vi "_API_BINANCE_GET_USDT_FUTURES_AccountInformation.vi"(0 "BinanceAPI in":refnum<class "BinanceAPI_.lvclass">, 11 "error in (no error)":errorcluster) -> (4 "BinanceAPI out":refnum<class "BinanceAPI_.lvclass">, 6 "data":T1, 14 "Data":string, 15 "error out":errorcluster)   [LabVIEW 2022 SP3, in "BinanceAPI_.lvclass"]
uses:
  BinanceAPI_.lvclass
  BinanceAPI_.lvclass/BinanceAPI_.ctl
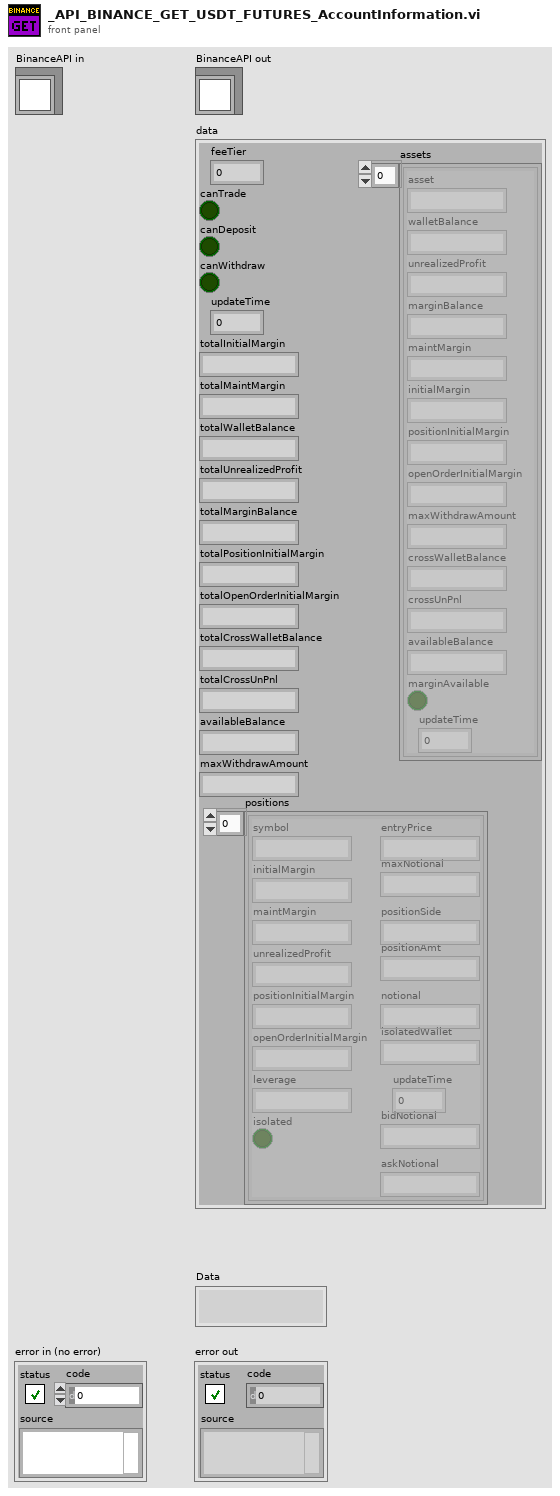
[diagram p1: front panel]
types:
  T1 = cluster{"feeTier":dbl, "canTrade":bool, "canDeposit":bool, "canWithdraw":bool, "updateTime":dbl, "totalInitialMargin":string, "totalMaintMargin":string, "totalWalletBalance":string, "totalUnrealizedProfit":string, "totalMarginBalance":string, "totalPositionInitialMargin":string, "totalOpenOrderInitialMargin":string, "totalCrossWalletBalance":string, "totalCrossUnPnl":string, "availableBalance":string, "maxWithdrawAmount":string, "assets":cluster{"asset":string, "walletBalance":string, "unrealizedProfit":string, "marginBalance":string, "maintMargin":string, "initialMargin":string, "positionInitialMargin":string, "openOrderInitialMargin":string, "maxWithdrawAmount":string, "crossWalletBalance":string, "crossUnPnl":string, "availableBalance":string, "marginAvailable":bool, "updateTime":dbl}[], "positions":cluster{"symbol":string, "initialMargin":string, "maintMargin":string, "unrealizedProfit":string, "positionInitialMargin":string, "openOrderInitialMargin":string, "leverage":string, "isolated":bool, "entryPrice":string, "maxNotional":string, "positionSide":string, "positionAmt":string, "notional":string, "isolatedWallet":string, "updateTime":dbl, "bidNotional":string, "askNotional":string}[]}
  T2 = enum16{"SPOT", "USDT_FUTURES", "COIN_FUTURES", "VANILLA"}
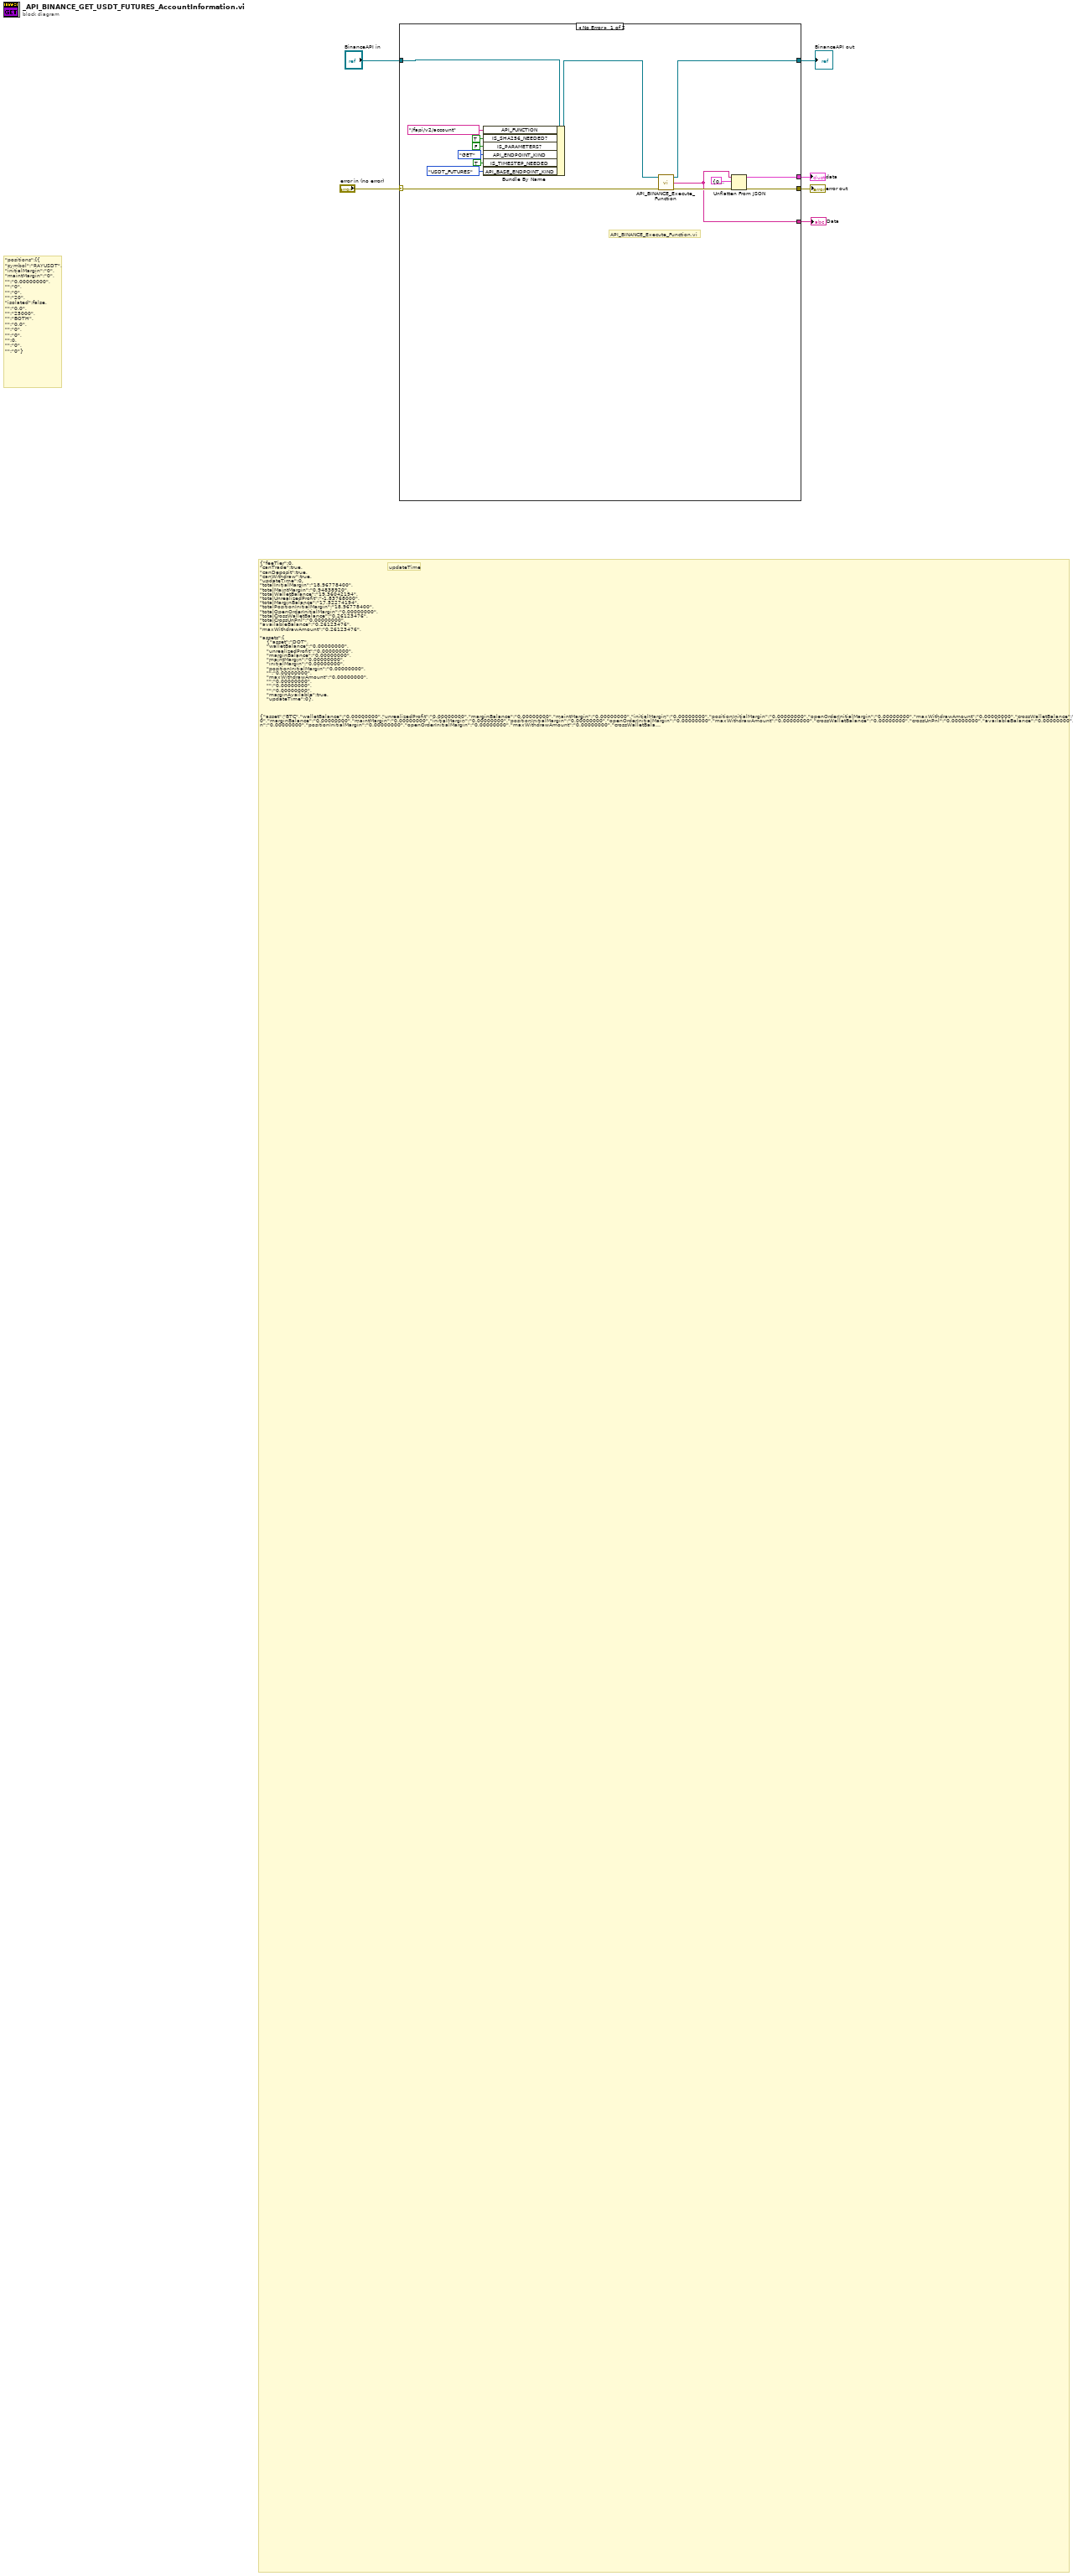
[diagram p0: block diagram]
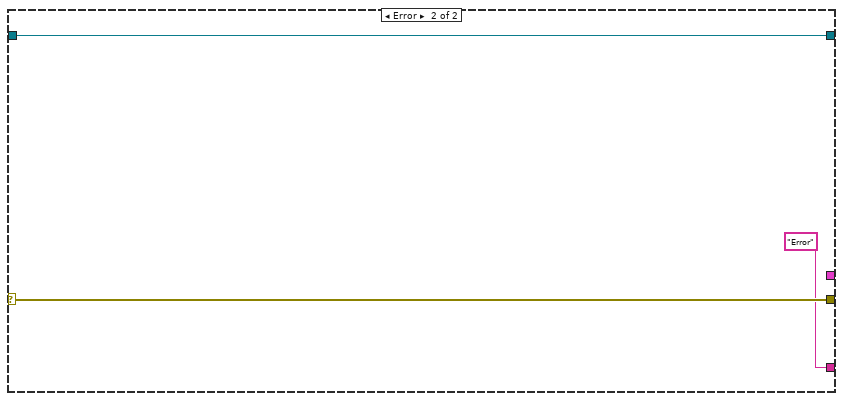
[diagram p2: hidden frame]
diagram:
  # "\"positions\":[{\n\"symbol\":\"RAYUSDT\",\n\"initialMargin\":\"0\",\n\"maintMargin\":\"0\",\n\"\":\"0.00000000\",\n\"\":\"0\",\n\"\":\"0\",\n\"\":\"20\",\n\"isolated\":false,\n\"\":\"0.0\",\n\"\":\"25000\",\n\"\":\"BOTH\",\n\"\":\"0.0\",\n\"\":\"0\",\n\"\":\"0\",\n\"\":0,\n\"\":\"0\",\n\"\":\"0\"}"
  # "updateTime"
  # "{\"feeTier\":0,\n\"canTrade\":true,\n\"canDeposit\":true,\n\"canWithdraw\":true,\n\"updateTime\":0,\n\"totalInitialMargin\":\"18.96778400\",\n\"totalMaintMargin\":\"0.94838920\",\n\"totalWalletBalance\":\"19.36042194\",\n\"totalUnrealizedProfit\":\"-1.83768000\",\n\"totalMarginBalance\":\"17.52274194\",\n\"totalPositionInitialMargin\":\"18.96778400\",\n\"totalOpenOrderInitialMargin\":\"0.00000000\",\n\"totalCrossWalletBalance\":\"0.26123476\",\n\"totalCrossUnPnl\":\"0.00000000\",\n\"availableBalance\":\"0.26123476\",\n\"maxWithdrawAmount\":\"0.26123476\",\n\n\"assets\":[\n    {\"asset\":\"DOT\",\n    \"walletBalance\":\"0.00000000\",\n    \"unrealizedProfit\":\"0.00000000\",\n    \"marginBalance\":\"0.00000000\",\n    \"maintMargin\":\"0.00000000\",\n    \"initialMargin\":\"0.00000000\",\n    \"positionInitialMargin\":\"0.00000000\",\n    \"\":\"0.00000000\",\n    \"maxWithdrawAmount\":\"0.00000000\",\n    \"\":\"0.00000000\",\n    \"\":\"0.00000000\",\n    \"\":\"0.00000000\",\n    \"marginAvailable\":true,\n    \"updateTime\":0},\n\n\n    {\"asset\":\"BTC\",\"walletBalance\":\"0.00000000\",\"unrealizedProfit\":\"0.00000000\",\"marginBalance\":\"0.00000000\",\"maintMargin\":\"0.00000000\",\"initialMargin\":\"0.00000000\",\"positionInitialMargin\":\"0.00000000\",\"openOrderInitialMargin\":\"0.00000000\",\"maxWithdrawAmount\":\"0.00000000\",\"crossWalletBalance\":\"0.00000000\",\"crossUnPnl\":\"0.00000000\",\"availableBalance\":\"0.00000000\",\"marginAvailable\":true,\"updateTime\":0},{\"asset\":\"SOL\",\"walletBalance\":\"0.00000000\",\"unrealizedProfit\":\"0.00000000\",\"marginBalance\":\"0.00000000\",\"maintMargin\":\"0.00000000\",\"initialMargin\":\"0.00000000\",\"positionInitialMargin\":\"0.00000000\",\"openOrderInitialMargin\":\"0.00000000\",\"maxWithdrawAmount\":\"0.00000000\",\"crossWalletBalance\":\"0.00000000\",\"crossUnPnl\":\"0.00000000\",\"availableBalance\":\"0.00000000\",\"marginAvailable\":true,\"updateTime\":0},{\"asset\":\"BNB\",\"walletBalance\":\"0.00000000\",\"unrealizedProfit\":\"0.00000000\",\"marginBalance\":\"0.00000000\",\"maintMargin\":\"0.00000000\",\"initialMargin\":\"0.00000000\",\"positionInitialMargin\":\"0.00000000\",\"openOrderInitialMargin\":\"0.00000000\",\"maxWithdrawAmount\":\"0.00000000\",\"crossWalletBalance\":\"0.00000000\",\"crossUnPnl\":\"0.00000000\",\"availableBalance\":\"0.00000000\",\"marginAvailable\":true,\"updateTime\":0},{\"asset\":\"ETH\",\"walletBalance\":\"0.00000000\",\"unrealizedProfit\":\"0.00000000\",\"marginBalance\":\"0.00000000\",\"maintMargin\":\"0.00000000\",\"initialMargin\":\"0.00000000\",\"positionInitialMargin\":\"0.00000000\",\"openOrderInitialMargin\":\"0.00000000\",\"maxWithdrawAmount\":\"0.00000000\",\"crossWalletBalance\":\"0.00000000\",\"crossUnPnl\":\"0.00000000\",\"availableBalance\":\"0.00000000\",\"marginAvailable\":true,\"updateTime\":0},{\"asset\":\"ADA\",\"walletBalance\":\"0.00000000\",\"unrealizedProfit\":\"0.00000000\",\"marginBalance\":\"0.00000000\",\"maintMargin\":\"0.00000000\",\"initialMargin\":\"0.00000000\",\"positionInitialMargin\":\"0.00000000\",\"openOrderInitialMargin\":\"0.00000000\",\"maxWithdrawAmount\":\"0.00000000\",\"crossWalletBalance\":\"0.00000000\",\"crossUnPnl\":\"0.00000000\",\"availableBalance\":\"0.00000000\",\"marginAvailable\":true,\"updateTime\":0},{\"asset\":\"USDT\",\"walletBalance\":\"19.36042194\",\"unrealizedProfit\":\"-1.83768000\",\"marginBalance\":\"17.52274194\",\"maintMargin\":\"0.94838920\",\"initialMargin\":\"18.96778400\",\"positionInitialMargin\":\"18.96778400\",\"openOrderInitialMargin\":\"0.00000000\",\"maxWithdrawAmount\":\"0.26123476\",\"crossWalletBalance\":\"0.26123476\",\"crossUnPnl\":\"0.00000000\",\"availableBalance\":\"0.26123476\",\"marginAvailable\":true,\"updateTime\":1658764800837},{\"asset\":\"XRP\",\"walletBalance\":\"0.00000000\",\"unrealizedProfit\":\"0.00000000\",\"marginBalance\":\"0.00000000\",\"maintMargin\":\"0.00000000\",\"initialMargin\":\"0.00000000\",\"positionInitialMargin\":\"0.00000000\",\"openOrderInitialMargin\":\"0.00000000\",\"maxWithdrawAmount\":\"0.00000000\",\"crossWalletBalance\":\"0.00000000\",\"crossUnPnl\":\"0.00000000\",\"availableBalance\":\"0.00000000\",\"marginAvailable\":true,\"updateTime\":0},{\"asset\":\"USDC\",\"walletBalance\":\"0.00000000\",\"unrealizedProfit\":\"0.00000000\",\"marginBalance\":\"0.00000000\",\"maintMargin\":\"0.00000000\",\"initialMargin\":\"0.00000000\",\"positionInitialMargin\":\"0.00000000\",\"openOrderInitialMargin\":\"0.00000000\",\"maxWithdrawAmount\":\"0.00000000\",\"crossWalletBalance\":\"0.00000000\",\"crossUnPnl\":\"0.00000000\",\"availableBalance\":\"0.00000000\",\"marginAvailable\":true,\"updateTime\":0},{\"asset\":\"BUSD\",\"walletBalance\":\"0.00000000\",\"unrealizedProfit\":\"0.00000000\",\"marginBalance\":\"0.00000000\",\"maintMargin\":\"0.00000000\",\"initialMargin\":\"0.00000000\",\"positionInitialMargin\":\"0.00000000\",\"openOrderInitialMargin\":\"0.00000000\",\"maxWithdrawAmount\":\"0.00000000\",\"crossWalletBalance\":\"0.00000000\",\"crossUnPnl\":\"0.00000000\",\"availableBalance\":\"0.00000000\",\"marginAvailable\":true,\"updateTime\":0}],\n\n\"positions\":[{\n\"symbol\":\"RAYUSDT\",\n\"initialMargin\":\"0\",\n\"maintMargin\":\"0\",\n\"unrealizedProfit\":\"0.00000000\",\n\"positionInitialMargin\":\"0\",\n\"openOrderInitialMargin\":\"0\",\n\"leverage\":\"20\",\n\"isolated\":false,\n\"entryPrice\":\"0.0\",\n\"maxNotional\":\"25000\",\n\"positionSide\":\"BOTH\",\n\"positionAmt\":\"0.0\",\n\"notional\":\"0\",\n\"isolatedWallet\":\"0\",\n\"updateTime\":0,\n\"bidNotional\":\"0\",\n\"askNotional\":\"0\"}\n\n,{\"symbol\":\"API3USDT\",\"initialMargin\":\"0\",\"maintMargin\":\"0\",\"unrealizedProfit\":\"0.00000000\",\"positionInitialMargin\":\"0\",\"openOrderInitialMargin\":\"0\",\"leverage\":\"20\",\"isolated\":false,\"entryPrice\":\"0.0\",\"maxNotional\":\"25000\",\"positionSide\":\"BOTH\",\"positionAmt\":\"0.0\",\"notional\":\"0\",\"isolatedWallet\":\"0\",\"updateTime\":0,\"bidNotional\":\"0\",\"askNotional\":\"0\"},{\"symbol\":\"SUSHIUSDT\",\"initialMargin\":\"0\",\"maintMargin\":\"0\",\"unrealizedProfit\":\"0.00000000\",\"positionInitialMargin\":\"0\",\"openOrderInitialMargin\":\"0\",\"leverage\":\"20\",\"isolated\":false,\"entryPrice\":\"0.0\",\"maxNotional\":\"25000\",\"positionSide\":\"BOTH\",\"positionAmt\":\"0\",\"notional\":\"0\",\"isolatedWallet\":\"0\",\"updateTime\":0,\"bidNotional\":\"0\",\"askNotional\":\"0\"},{\"symbol\":\"CVCUSDT\",\"initialMargin\":\"0\",\"maintMargin\":\"0\",\"unrealizedProfit\":\"0.00000000\",\"positionInitialMargin\":\"0\",\"openOrderInitialMargin\":\"0\",\"leverage\":\"20\",\"isolated\":false,\"entryPrice\":\"0.0\",\"maxNotional\":\"25000\",\"positionSide\":\"BOTH\",\"positionAmt\":\"0\",\"notional\":\"0\",\"isolatedWallet\":\"0\",\"updateTime\":0,\"bidNotional\":\"0\",\"askNotional\":\"0\"},{\"symbol\":\"BTSUSDT\",\"initialMargin\":\"0\",\"maintMargin\":\"0\",\"unrealizedProfit\":\"0.00000000\",\"positionInitialMargin\":\"0\",\"openOrderInitialMargin\":\"0\",\"leverage\":\"20\",\"isolated\":false,\"entryPrice\":\"0.0\",\"maxNotional\":\"25000\",\"positionSide\":\"BOTH\",\"positionAmt\":\"0\",\"notional\":\"0\",\"isolatedWallet\":\"0\",\"updateTime\":0,\"bidNotional\":\"0\",\"askNotional\":\"0\"},{\"symbol\":\"FTMBUSD\",\"initialMargin\":\"0\",\"maintMargin\":\"0\",\"unrealizedProfit\":\"0.00000000\",\"positionInitialMargin\":\"0\",\"openOrderInitialMargin\":\"0\",\"leverage\":\"20\",\"isolated\":false,\"entryPrice\":\"0.0\",\"maxNotional\":\"25000\",\"positionSide\":\"BOTH\",\"positionAmt\":\"0\",\"notional\":\"0\",\"isolatedWallet\":\"0\",\"updateTime\":0,\"bidNotional\":\"0\",\"askNotional\":\"0\"},{\"symbol\":\"LINKBUSD\",\"initialMargin\":\"0\",\"maintMargin\":\"0\",\"unrealizedProfit\":\"0.00000000\",\"positionInitialMargin\":\"0\",\"openOrderInitialMargin\":\"0\",\"leverage\":\"20\",\"isolated\":false,\"entryPrice\":\"0.0\",\"maxNotional\":\"25000\",\"positionSide\":\"BOTH\",\"positionAmt\":\"0.0\",\"notional\":\"0\",\"isolatedWallet\":\"0\",\"updateTime\":0,\"bidNotional\":\"0\",\"askNotional\":\"0\"},{\"symbol\":\"SANDBUSD\",\"initialMargin\":\"0\",\"maintMargin\":\"0\",\"unrealizedProfit\":\"0.00000000\",\"positionInitialMargin\":\"0\",\"openOrderInitialMargin\":\"0\",\"leverage\":\"20\",\"isolated\":false,\"entryPrice\":\"0.0\",\"maxNotional\":\"25000\",\"positionSide\":\"BOTH\",\"positionAmt\":\"0.0\",\"notional\":\"0\",\"isolatedWallet\":\"0\",\"updateTime\":0,\"bidNotional\":\"0\",\"askNotional\":\"0\"},{\"symbol\":\"HOTUSDT\",\"initialMargin\":\"0\",\"maintMargin\":\"0\",\"unrealizedProfit\":\"0.00000000\",\"positionInitialMargin\":\"0\",\"openOrderInitialMargin\":\"0\",\"leverage\":\"20\",\"isolated\":false,\"entryPrice\":\"0.0\",\"maxNotional\":\"25000\",\"positionSide\":\"BOTH\",\"positionAmt\":\"0\",\"notional\":\"0\",\"isolatedWallet\":\"0\",\"updateTime\":0,\"bidNotional\":\"0\",\"askNotional\":\"0\"},{\"symbol\":\"TRXBUSD\",\"initialMargin\":\"0\",\"maintMargin\":\"0\",\"unrealizedProfit\":\"0.00000000\",\"positionInitialMargin\":\"0\",\"openOrderInitialMargin\":\"0\",\"leverage\":\"20\",\"isolated\":false,\"entryPrice\":\"0.0\",\"maxNotional\":\"25000\",\"positionSide\":\"BOTH\",\"positionAmt\":\"0\",\"notional\":\"0\",\"isolatedWallet\":\"0\",\"updateTime\":0,\"bidNotional\":\"0\",\"askNotional\":\"0\"},{\"symbol\":\"ZRXUSDT\",\"initialMargin\":\"0\",\"maintMargin\":\"0\",\"unrealizedProfit\":\"0.00000000\",\"positionInitialMargin\":\"0\",\"openOrderInitialMargin\":\"0\",\"leverage\":\"20\",\"isolated\":false,\"entryPrice\":\"0.0\",\"maxNotional\":\"25000\",\"positionSide\":\"BOTH\",\"positionAmt\":\"0.0\",\"notional\":\"0\",\"isolatedWallet\":\"0\",\"updateTime\":0,\"bidNotional\":\"0\",\"askNotional\":\"0\"},{\"symbol\":\"QTUMUSDT\",\"initialMargin\":\"0\",\"maintMargin\":\"0\",\"unrealizedProfit\":\"0.00000000\",\"positionInitialMargin\":\"0\",\"openOrderInitialMargin\":\"0\",\"leverage\":\"20\",\"isolated\":false,\"entryPrice\":\"0.0\",\"maxNotional\":\"25000\",\"positionSide\":\"BOTH\",\"positionAmt\":\"0.0\",\"notional\":\"0\",\"isolatedWallet\":\"0\",\"updateTime\":0,\"bidNotional\":\"0\",\"askNotional\":\"0\"},{\"symbol\":\"IOTAUSDT\",\"initialMargin\":\"0\",\"maintMargin\":\"0\",\"unrealizedProfit\":\"0.00000000\",\"positionInitialMargin\":\"0\",\"openOrderInitialMargin\":\"0\",\"leverage\":\"20\",\"isolated\":false,\"entryPrice\":\"0.0\",\"maxNotional\":\"25000\",\"positionSide\":\"BOTH\",\"positionAmt\":\"0.0\",\"notional\":\"0\",\"isolatedWallet\":\"0\",\"updateTime\":0,\"bidNotional\":\"0\",\"askNotional\":\"0\"},{\"symbol\":\"BTCBUSD\",\"initialMargin\":\"0\",\"maintMargin\":\"0\",\"unrealizedProfit\":\"0.00000000\",\"positionInitialMargin\":\"0\",\"openOrderInitialMargin\":\"0\",\"leverage\":\"20\",\"isolated\":false,\"entryPrice\":\"0.0\",\"maxNotional\":\"1000000\",\"positionSide\":\"BOTH\",\"positionAmt\":\"0.000\",\"notional\":\"0\",\"isolatedWallet\":\"0\",\"updateTime\":0,\"bidNotional\":\"0\",\"askNotional\":\"0\"},{\"symbol\":\"WAVESUSDT\",\"initialMargin\":\"0\",\"maintMargin\":\"0\",\"unrealizedProfit\":\"0.00000000\",\"positionInitialMargin\":\"0\",\"openOrderInitialMargin\":\"0\",\"leverage\":\"50\",\"isolated\":false,\"entryPrice\":\"0.0\",\"maxNotional\":\"5000\",\"positionSide\":\"BOTH\",\"positionAmt\":\"0.0\",\"notional\":\"0\",\"isolatedWallet\":\"0\",\"updateTime\":1655896560449,\"bidNotional\":\"0\",\"askNotional\":\"0\"},{\"symbol\":\"ADAUSDT\",\"initialMargin\":\"0\",\"maintMargin\":\"0\",\"unrealizedProfit\":\"0.00000000\",\"positionInitialMargin\":\"0\",\"openOrderInitialMargin\":\"0\",\"leverage\":\"20\",\"isolated\":false,\"entryPrice\":\"0.0\",\"maxNotional\":\"250000\",\"positionSide\":\"BOTH\",\"positionAmt\":\"0\",\"notional\":\"0\",\"isolatedWallet\":\"0\",\"updateTime\":0,\"bidNotional\":\"0\",\"askNotional\":\"0\"},{\"symbol\":\"LITUSDT\",\"initialMargin\":\"0\",\"maintMargin\":\"0\",\"unrealizedProfit\":\"0.00000000\",\"positionInitialMargin\":\"0\",\"openOrderInitialMargin\":\"0\",\"leverage\":\"20\",\"isolated\":false,\"entryPrice\":\"0.0\",\"maxNotional\":\"25000\",\"positionSide\":\"BOTH\",\"positionAmt\":\"0.0\",\"notional\":\"0\",\"isolatedWallet\":\"0\",\"updateTime\":0,\"bidNotional\":\"0\",\"askNotional\":\"0\"},{\"symbol\":\"XTZUSDT\",\"initialMargin\":\"0\",\"maintMargin\":\"0\",\"unrealizedProfit\":\"0.00000000\",\"positionInitialMargin\":\"0\",\"openOrderInitialMargin\":\"0\",\"leverage\":\"20\",\"isolated\":false,\"entryPrice\":\"0.0\",\"maxNotional\":\"250000\",\"positionSide\":\"BOTH\",\"positionAmt\":\"0.0\",\"notional\":\"0\",\"isolatedWallet\":\"0\",\"updateTime\":0,\"bidNotional\":\"0\",\"askNotional\":\"0\"},{\"symbol\":\"BNBUSDT\",\"initialMargin\":\"0\",\"maintMargin\":\"0\",\"unrealizedProfit\":\"0.00000000\",\"positionInitialMargin\":\"0\",\"openOrderInitialMargin\":\"0\",\"leverage\":\"75\",\"isolated\":true,\"entryPrice\":\"0.0\",\"maxNotional\":\"10000\",\"positionSide\":\"BOTH\",\"positionAmt\":\"0.00\",\"notional\":\"0\",\"isolatedWallet\":\"0\",\"updateTime\":1653521652424,\"bidNotional\":\"0\",\"askNotional\":\"0\"},{\"symbol\":\"DARUSDT\",\"initialMargin\":\"0\",\"maintMargin\":\"0\",\"unrealizedProfit\":\"0.00000000\",\"positionInitialMargin\":\"0\",\"openOrderInitialMargin\":\"0\",\"leverage\":\"20\",\"isolated\":false,\"entryPrice\":\"0.0\",\"maxNotional\":\"25000\",\"positionSide\":\"BOTH\",\"positionAmt\":\"0.0\",\"notional\":\"0\",\"isolatedWallet\":\"0\",\"updateTime\":0,\"bidNotional\":\"0\",\"askNotional\":\"0\"},{\"symbol\":\"HNTUSDT\",\"initialMargin\":\"0\",\"maintMargin\":\"0\",\"unrealizedProfit\":\"0.00000000\",\"positionInitialMargin\":\"0\",\"openOrderInitialMargin\":\"0\",\"leverage\":\"20\",\"isolated\":false,\"entryPrice\":\"0.0\",\"maxNotional\":\"25000\",\"positionSide\":\"BOTH\",\"positionAmt\":\"0\",\"notional\":\"0\",\"isolatedWallet\":\"0\",\"updateTime\":0,\"bidNotional\":\"0\",\"askNotional\":\"0\"},{\"symbol\":\"ETCUSDT\",\"initialMargin\":\"0\",\"maintMargin\":\"0\",\"unrealizedProfit\":\"0.00000000\",\"positionInitialMargin\":\"0\",\"openOrderInitialMargin\":\"0\",\"leverage\":\"20\",\"isolated\":false,\"entryPrice\":\"0.0\",\"maxNotional\":\"250000\",\"positionSide\":\"BOTH\",\"positionAmt\":\"0.00\",\"notional\":\"0\",\"isolatedWallet\":\"0\",\"updateTime\":0,\"bidNotional\":\"0\",\"askNotional\":\"0\"},{\"symbol\":\"XMRUSDT\",\"initialMargin\":\"0\",\"maintMargin\":\"0\",\"unrealizedProfit\":\"0.00000000\",\"positionInitialMargin\":\"0\",\"openOrderInitialMargin\":\"0\",\"leverage\":\"20\",\"isolated\":false,\"entryPrice\":\"0.0\",\"maxNotional\":\"250000\",\"positionSide\":\"BOTH\",\"positionAmt\":\"0.000\",\"notional\":\"0\",\"isolatedWallet\":\"0\",\"updateTime\":0,\"bidNotional\":\"0\",\"askNotional\":\"0\"},{\"symbol\":\"YFIUSDT\",\"initialMargin\":\"0\",\"maintMargin\":\"0\",\"unrealizedProfit\":\"0.00000000\",\"positionInitialMargin\":\"0\",\"openOrderInitialMargin\":\"0\",\"leverage\":\"20\",\"isolated\":false,\"entryPrice\":\"0.0\",\"maxNotional\":\"25000\",\"positionSide\":\"BOTH\",\"positionAmt\":\"0.000\",\"notional\":\"0\",\"isolatedWallet\":\"0\",\"updateTime\":0,\"bidNotional\":\"0\",\"askNotional\":\"0\"},{\"symbol\":\"FTTBUSD\",\"initialMargin\":\"0\",\"maintMargin\":\"0\",\"unrealizedProfit\":\"0.00000000\",\"positionInitialMargin\":\"0\",\"openOrderInitialMargin\":\"0\",\"leverage\":\"20\",\"isolated\":false,\"entryPrice\":\"0.0\",\"maxNotional\":\"100000\",\"positionSide\":\"BOTH\",\"positionAmt\":\"0.0\",\"notional\":\"0\",\"isolatedWallet\":\"0\",\"updateTime\":0,\"bidNotional\":\"0\",\"askNotional\":\"0\"},{\"symbol\":\"ETHUSDT\",\"initialMargin\":\"18.96778400\",\"maintMargin\":\"0.94838920\",\"unrealizedProfit\":\"-1.83768000\",\"positionInitialMargin\":\"18.96778400\",\"openOrderInitialMargin\":\"0\",\"leverage\":\"10\",\"isolated\":true,\"entryPrice\":\"1544.48\",\"maxNotional\":\"4000000\",\"positionSide\":\"BOTH\",\"positionAmt\":\"0.124\",\"notional\":\"189.67784000\",\"isolatedWallet\":\"19.09918718\",\"updateTime\":1658764800837,\"bidNotional\":\"0\",\"askNotional\":\"0\"},{\"symbol\":\"ALICEUSDT\",\"initialMargin\":\"0\",\"maintMargin\":\"0\",\"unrealizedProfit\":\"0.00000000\",\"positionInitialMargin\":\"0\",\"openOrderInitialMargin\":\"0\",\"leverage\":\"20\",\"isolated\":false,\"entryPrice\":\"0.0\",\"maxNotional\":\"25000\",\"positionSide\":\"BOTH\",\"positionAmt\":\"0.0\",\"notional\":\"0\",\"isolatedWallet\":\"0\",\"updateTime\":0,\"bidNotional\":\"0\",\"askNotional\":\"0\"},{\"symbol\":\"ALPHAUSDT\",\"initialMargin\":\"0\",\"maintMargin\":\"0\",\"unrealizedProfit\":\"0.00000000\",\"positionInitialMargin\":\"0\",\"openOrderInitialMargin\":\"0\",\"leverage\":\"20\",\"isolated\":false,\"entryPrice\":\"0.0\",\"maxNotional\":\"25000\",\"positionSide\":\"BOTH\",\"positionAmt\":\"0\",\"notional\":\"0\",\"isolatedWallet\":\"0\",\"updateTime\":0,\"bidNotional\":\"0\",\"askNotional\":\"0\"},{\"symbol\":\"WOOUSDT\",\"initialMargin\":\"0\",\"maintMargin\":\"0\",\"unrealizedProfit\":\"0.00000000\",\"positionInitialMargin\":\"0\",\"openOrderInitialMargin\":\"0\",\"leverage\":\"20\",\"isolated\":false,\"entryPrice\":\"0.0\",\"maxNotional\":\"25000\",\"positionSide\":\"BOTH\",\"positionAmt\":\"0\",\"notional\":\"0\",\"isolatedWallet\":\"0\",\"updateTime\":0,\"bidNotional\":\"0\",\"askNotional\":\"0\"},{\"symbol\":\"SFPUSDT\",\"initialMargin\":\"0\",\"maintMargin\":\"0\",\"unrealizedProfit\":\"0.00000000\",\"positionInitialMargin\":\"0\",\"openOrderInitialMargin\":\"0\",\"leverage\":\"20\",\"isolated\":false,\"entryPrice\":\"0.0\",\"maxNotional\":\"25000\",\"positionSide\":\"BOTH\",\"positionAmt\":\"0\",\"notional\":\"0\",\"isolatedWallet\":\"0\",\"updateTime\":0,\"bidNotional\":\"0\",\"askNotional\":\"0\"},{\"symbol\":\"REEFUSDT\",\"initialMargin\":\"0\",\"maintMargin\":\"0\",\"unrealizedProfit\":\"0.00000000\",\"positionInitialMargin\":\"0\",\"openOrderInitialMargin\":\"0\",\"leverage\":\"20\",\"isolated\":false,\"entryPrice\":\"0.0\",\"maxNotional\":\"25000\",\"positionSide\":\"BOTH\",\"positionAmt\":\"0\",\"notional\":\"0\",\"isolatedWallet\":\"0\",\"updateTime\":0,\"bidNotional\":\"0\",\"askNotional\":\"0\"},{\"symbol\":\"BATUSDT\",\"initialMargin\":\"0\",\"maintMargin\":\"0\",\"unrealizedProfit\":\"0.00000000\",\"positionInitialMargin\":\"0\",\"openOrderInitialMargin\":\"0\",\"leverage\":\"20\",\"isolated\":false,\"entryPrice\":\"0.0\",\"maxNotional\":\"25000\",\"positionSide\":\"BOTH\",\"positionAmt\":\"0.0\",\"notional\":\"0\",\"isolatedWallet\":\"0\",\"updateTime\":0,\"bidNotional\":\"0\",\"askNotional\":\"0\"},{\"symbol\":\"DOGEUSDT\",\"initialMargin\":\"0\",\"maintMargin\":\"0\",\"unrealizedProfit\":\"0.00000000\",\"positionInitialMargin\":\"0\",\"openOrderInitialMargin\":\"0\",\"leverage\":\"50\",\"isolated\":true,\"entryPrice\":\"0.0\",\"maxNotional\":\"50000\",\"positionSide\":\"BOTH\",\"positionAmt\":\"0\",\"notional\":\"0\",\"isolatedWallet\":\"0\",\"updateTime\":1653473172278,\"bidNotional\":\"0\",\"askNotional\":\"0\"},{\"symbol\":\"TRXUSDT\",\"initialMargin\":\"0\",\"maintMargin\":\"0\",\"unrealizedProfit\":\"0.00000000\",\"positionInitialMargin\":\"0\",\"openOrderInitialMargin\":\"0\",\"leverage\":\"20\",\"isolated\":false,\"entryPrice\":\"0.0\",\"maxNotional\":\"250000\",\"positionSide\":\"BOTH\",\"positionAmt\":\"0\",\"notional\":\"0\",\"isolatedWallet\":\"0\",\"updateTime\":0,\"bidNotional\":\"0\",\"askNotional\":\"0\"},{\"symbol\":\"RLCUSDT\",\"initialMargin\":\"0\",\"maintMargin\":\"0\",\"unrealizedProfit\":\"0.00000000\",\"positionInitialMargin\":\"0\",\"openOrderInitialMargin\":\"0\",\"leverage\":\"20\",\"isolated\":false,\"entryPrice\":\"0.0\",\"maxNotional\":\"25000\",\"positionSide\":\"BOTH\",\"positionAmt\":\"0.0\",\"notional\":\"0\",\"isolatedWallet\":\"0\",\"updateTime\":0,\"bidNotional\":\"0\",\"askNotional\":\"0\"},{\"symbol\":\"BTCSTUSDT\",\"initialMargin\":\"0\",\"maintMargin\":\"0\",\"unrealizedProfit\":\"0.00000000\",\"positionInitialMargin\":\"0\",\"openOrderInitialMargin\":\"0\",\"leverage\":\"20\",\"isolated\":false,\"entryPrice\":\"0.0\",\"maxNotional\":\"25000\",\"positionSide\":\"BOTH\",\"positionAmt\":\"0.0\",\"notional\":\"0\",\"isolatedWallet\":\"0\",\"updateTime\":0,\"bidNotional\":\"0\",\"askNotional\":\"0\"},{\"symbol\":\"STORJUSDT\",\"initialMargin\":\"0\",\"maintMargin\":\"0\",\"unrealizedProfit\":\"0.00000000\",\"positionInitialMargin\":\"0\",\"openOrderInitialMargin\":\"0\",\"leverage\":\"20\",\"isolated\":false,\"entryPrice\":\"0.0\",\"maxNotional\":\"25000\",\"positionSide\":\"BOTH\",\"positionAmt\":\"0\",\"notional\":\"0\",\"isolatedWallet\":\"0\",\"updateTime\":0,\"bidNotional\":\"0\",\"askNotional\":\"0\"},{\"symbol\":\"SNXUSDT\",\"initialMargin\":\"0\",\"maintMargin\":\"0\",\"unrealizedProfit\":\"0.00000000\",\"positionInitialMargin\":\"0\",\"openOrderInitialMargin\":\"0\",\"leverage\":\"20\",\"isolated\":false,\"entryPrice\":\"0.0\",\"maxNotional\":\"25000\",\"positionSide\":\"BOTH\",\"positionAmt\":\"0.0\",\"notional\":\"0\",\"isolatedWallet\":\"0\",\"updateTime\":0,\"bidNotional\":\"0\",\"askNotional\":\"0\"},{\"symbol\":\"1000XECUSDT\",\"initialMargin\":\"0\",\"maintMargin\":\"0\",\"unrealizedProfit\":\"0.00000000\",\"positionInitialMargin\":\"0\",\"openOrderInitialMargin\":\"0\",\"leverage\":\"20\",\"isolated\":false,\"entryPrice\":\"0.0\",\"maxNotional\":\"25000\",\"positionSide\":\"BOTH\",\"positionAmt\":\"0\",\"notional\":\"0\",\"isolatedWallet\":\"0\",\"updateTime\":0,\"bidNotional\":\"0\",\"askNotional\":\"0\"},{\"symbol\":\"DOTBUSD\",\"initialMargin\":\"0\",\"maintMargin\":\"0\",\"unrealizedProfit\":\"0.00000000\",\"positionInitialMargin\":\"0\",\"openOrderInitialMargin\":\"0\",\"leverage\":\"20\",\"isolated\":false,\"entryPrice\":\"0.0\",\"maxNotional\":\"25000\",\"positionSide\":\"BOTH\",\"positionAmt\":\"0.0\",\"notional\":\"0\",\"isolatedWallet\":\"0\",\"updateTime\":0,\"bidNotional\":\"0\",\"askNotional\":\"0\"},{\"symbol\":\"AUDIOUSDT\",\"initialMargin\":\"0\",\"maintMargin\":\"0\",\"unrealizedProfit\":\"0.00000000\",\"positionInitialMargin\":\"0\",\"openOrderInitialMargin\":\"0\",\"leverage\":\"20\",\"isolated\":false,\"entryPrice\":\"0.0\",\"maxNotional\":\"25000\",\"positionSide\":\"BOTH\",\"positionAmt\":\"0\",\"notional\":\"0\",\"isolatedWallet\":\"0\",\"updateTime\":0,\"bidNotional\":\"0\",\"askNotional\":\"0\"},{\"symbol\":\"NEARBUSD\",\"initialMargin\":\"0\",\"maintMargin\":\"0\",\"unrealizedProfit\":\"0.00000000\",\"positionInitialMargin\":\"0\",\"openOrderInitialMargin\":\"0\",\"leverage\":\"20\",\"isolated\":false,\"entryPrice\":\"0.0\",\"maxNotional\":\"25000\",\"positionSide\":\"BOTH\",\"positionAmt\":\"0.0\",\"notional\":\"0\",\"isolatedWallet\":\"0\",\"updateTime\":0,\"bidNotional\":\"0\",\"askNotional\":\"0\"},{\"symbol\":\"XLMUSDT\",\"initialMargin\":\"0\",\"maintMargin\":\"0\",\"unrealizedProfit\":\"0.00000000\",\"positionInitialMargin\":\"0\",\"openOrderInitialMargin\":\"0\",\"leverage\":\"20\",\"isolated\":false,\"entryPrice\":\"0.0\",\"maxNotional\":\"250000\",\"positionSide\":\"BOTH\",\"positionAmt\":\"0\",\"notional\":\"0\",\"isolatedWallet\":\"0\",\"updateTime\":0,\"bidNotional\":\"0\",\"askNotional\":\"0\"},{\"symbol\":\"APEBUSD\",\"initialMargin\":\"0\",\"maintMargin\":\"0\",\"unrealizedProfit\":\"0.00000000\",\"positionInitialMargin\":\"0\",\"openOrderInitialMargin\":\"0\",\"leverage\":\"20\",\"isolated\":false,\"entryPrice\":\"0.0\",\"maxNotional\":\"25000\",\"positionSide\":\"BOTH\",\"positionAmt\":\"0.0\",\"notional\":\"0\",\"isolatedWallet\":\"0\",\"updateTime\":0,\"bidNotional\":\"0\",\"askNotional\":\"0\"},{\"symbol\":\"IOTXUSDT\",\"initialMargin\":\"0\",\"maintMargin\":\"0\",\"unrealizedProfit\":\"0.00000000\",\"positionInitialMargin\":\"0\",\"openOrderInitialMargin\":\"0\",\"leverage\":\"20\",\"isolated\":false,\"entryPrice\":\"0.0\",\"maxNotional\":\"25000\",\"positionSide\":\"BOTH\",\"positionAmt\":\"0\",\"notional\":\"0\",\"isolatedWallet\":\"0\",\"updateTime\":0,\"bidNotional\":\"0\",\"askNotional\":\"0\"},{\"symbol\":\"NEOUSDT\",\"initialMargin\":\"0\",\"maintMargin\":\"0\",\"unrealizedProfit\":\"0.00000000\",\"positionInitialMargin\":\"0\",\"openOrderInitialMargin\":\"0\",\"leverage\":\"20\",\"isolated\":false,\"entryPrice\":\"0.0\",\"maxNotional\":\"25000\",\"positionSide\":\"BOTH\",\"positionAmt\":\"0.00\",\"notional\":\"0\",\"isolatedWallet\":\"0\",\"updateTime\":0,\"bidNotional\":\"0\",\"askNotional\":\"0\"},{\"symbol\":\"UNFIUSDT\",\"initialMargin\":\"0\",\"maintMargin\":\"0\",\"unrealizedProfit\":\"0.00000000\",\"positionInitialMargin\":\"0\",\"openOrderInitialMargin\":\"0\",\"leverage\":\"20\",\"isolated\":false,\"entryPrice\":\"0.0\",\"maxNotional\":\"25000\",\"positionSide\":\"BOTH\",\"positionAmt\":\"0.0\",\"notional\":\"0\",\"isolatedWallet\":\"0\",\"updateTime\":0,\"bidNotional\":\"0\",\"askNotional\":\"0\"},{\"symbol\":\"SANDUSDT\",\"initialMargin\":\"0\",\"maintMargin\":\"0\",\"unrealizedProfit\":\"0.00000000\",\"positionInitialMargin\":\"0\",\"openOrderInitialMargin\":\"0\",\"leverage\":\"3\",\"isolated\":false,\"entryPrice\":\"0.0\",\"maxNotional\":\"1000000\",\"positionSide\":\"BOTH\",\"positionAmt\":\"0\",\"notional\":\"0\",\"isolatedWallet\":\"0\",\"updateTime\":1638400731902,\"bidNotional\":\"0\",\"askNotional\":\"0\"},{\"symbol\":\"DASHUSDT\",\"initialMargin\":\"0\",\"maintMargin\":\"0\",\"unrealizedProfit\":\"0.00000000\",\"positionInitialMargin\":\"0\",\"openOrderInitialMargin\":\"0\",\"leverage\":\"20\",\"isolated\":false,\"entryPrice\":\"0.0\",\"maxNotional\":\"25000\",\"positionSide\":\"BOTH\",\"positionAmt\":\"0.000\",\"notional\":\"0\",\"isolatedWallet\":\"0\",\"updateTime\":0,\"bidNotional\":\"0\",\"askNotional\":\"0\"},{\"symbol\":\"KAVAUSDT\",\"initialMargin\":\"0\",\"maintMargin\":\"0\",\"unrealizedProfit\":\"0.00000000\",\"positionInitialMargin\":\"0\",\"openOrderInitialMargin\":\"0\",\"leverage\":\"20\",\"isolated\":false,\"entryPrice\":\"0.0\",\"maxNotional\":\"25000\",\"positionSide\":\"BOTH\",\"positionAmt\":\"0.0\",\"notional\":\"0\",\"isolatedWallet\":\"0\",\"updateTime\":0,\"bidNotional\":\"0\",\"askNotional\":\"0\"},{\"symbol\":\"RUNEUSDT\",\"initialMargin\":\"0\",\"maintMargin\":\"0\",\"unrealizedProfit\":\"0.00000000\",\"positionInitialMargin\":\"0\",\"openOrderInitialMargin\":\"0\",\"leverage\":\"20\",\"isolated\":false,\"entryPrice\":\"0.0\",\"maxNotional\":\"25000\",\"positionSide\":\"BOTH\",\"positionAmt\":\"0\",\"notional\":\"0\",\"isolatedWallet\":\"0\",\"updateTime\":0,\"bidNotional\":\"0\",\"askNotional\":\"0\"},{\"symbol\":\"APEUSDT\",\"initialMargin\":\"0\",\"maintMargin\":\"0\",\"unrealizedProfit\":\"0.00000000\",\"positionInitialMargin\":\"0\",\"openOrderInitialMargin\":\"0\",\"leverage\":\"20\",\"isolated\":false,\"entryPrice\":\"0.0\",\"maxNotional\":\"150000\",\"positionSide\":\"BOTH\",\"positionAmt\":\"0\",\"notional\":\"0\",\"isolatedWallet\":\"0\",\"updateTime\":0,\"bidNotional\":\"0\",\"askNotional\":\"0\"},{\"symbol\":\"CTKUSDT\",\"initialMargin\":\"0\",\"maintMargin\":\"0\",\"unrealizedProfit\":\"0.00000000\",\"positionInitialMargin\":\"0\",\"openOrderInitialMargin\":\"0\",\"leverage\":\"20\",\"isolated\":false,\"entryPrice\":\"0.0\",\"maxNotional\":\"25000\",\"positionSide\":\"BOTH\",\"positionAmt\":\"0\",\"notional\":\"0\",\"isolatedWallet\":\"0\",\"updateTime\":0,\"bidNotional\":\"0\",\"askNotional\":\"0\"},{\"symbol\":\"LINKUSDT\",\"initialMargin\":\"0\",\"maintMargin\":\"0\",\"unrealizedProfit\":\"0.00000000\",\"positionInitialMargin\":\"0\",\"openOrderInitialMargin\":\"0\",\"leverage\":\"20\",\"isolated\":false,\"entryPrice\":\"0.0\",\"maxNotional\":\"250000\",\"positionSide\":\"BOTH\",\"positionAmt\":\"0.00\",\"notional\":\"0\",\"isolatedWallet\":\"0\",\"updateTime\":0,\"bidNotional\":\"0\",\"askNotional\":\"0\"},{\"symbol\":\"CELRUSDT\",\"initialMargin\":\"0\",\"maintMargin\":\"0\",\"unrealizedProfit\":\"0.00000000\",\"positionInitialMargin\":\"0\",\"openOrderInitialMargin\":\"0\",\"leverage\":\"20\",\"isolated\":false,\"entryPrice\":\"0.0\",\"maxNotional\":\"25000\",\"positionSide\":\"BOTH\",\"positionAmt\":\"0\",\"notional\":\"0\",\"isolatedWallet\":\"0\",\"updateTime\":0,\"bidNotional\":\"0\",\"askNotional\":\"0\"},{\"symbol\":\"BNXUSDT\",\"initialMargin\":\"0\",\"maintMargin\":\"0\",\"unrealizedProfit\":\"0.00000000\",\"positionInitialMargin\":\"0\",\"openOrderInitialMargin\":\"0\",\"leverage\":\"20\",\"isolated\":false,\"entryPrice\":\"0.0\",\"maxNotional\":\"150000\",\"positionSide\":\"BOTH\",\"positionAmt\":\"0.0\",\"notional\":\"0\",\"isolatedWallet\":\"0\",\"updateTime\":0,\"bidNotional\":\"0\",\"askNotional\":\"0\"},{\"symbol\":\"CVXBUSD\",\"initialMargin\":\"0\",\"maintMargin\":\"0\",\"unrealizedProfit\":\"0.00000000\",\"positionInitialMargin\":\"0\",\"openOrderInitialMargin\":\"0\",\"leverage\":\"20\",\"isolated\":false,\"entryPrice\":\"0.0\",\"maxNotional\":\"25000\",\"positionSide\":\"BOTH\",\"positionAmt\":\"0.0\",\"notional\":\"0\",\"isolatedWallet\":\"0\",\"updateTime\":0,\"bidNotional\":\"0\",\"askNotional\":\"0\"},{\"symbol\":\"OPUSDT\",\"initialMargin\":\"0\",\"maintMargin\":\"0\",\"unrealizedProfit\":\"0.00000000\",\"positionInitialMargin\":\"0\",\"openOrderInitialMargin\":\"0\",\"leverage\":\"20\",\"isolated\":false,\"entryPrice\":\"0.0\",\"maxNotional\":\"25000\",\"positionSide\":\"BOTH\",\"positionAmt\":\"0.0\",\"notional\":\"0\",\"isolatedWallet\":\"0\",\"updateTime\":0,\"bidNotional\":\"0\",\"askNotional\":\"0\"},{\"symbol\":\"RSRUSDT\",\"initialMargin\":\"0\",\"maintMargin\":\"0\",\"unrealizedProfit\":\"0.00000000\",\"positionInitialMargin\":\"0\",\"openOrderInitialMargin\":\"0\",\"leverage\":\"20\",\"isolated\":false,\"entryPrice\":\"0.0\",\"maxNotional\":\"25000\",\"positionSide\":\"BOTH\",\"positionAmt\":\"0\",\"notional\":\"0\",\"isolatedWallet\":\"0\",\"updateTime\":0,\"bidNotional\":\"0\",\"askNotional\":\"0\"},{\"symbol\":\"ADABUSD\",\"initialMargin\":\"0\",\"maintMargin\":\"0\",\"unrealizedProfit\":\"0.00000000\",\"positionInitialMargin\":\"0\",\"openOrderInitialMargin\":\"0\",\"leverage\":\"20\",\"isolated\":false,\"entryPrice\":\"0.0\",\"maxNotional\":\"100000\",\"positionSide\":\"BOTH\",\"positionAmt\":\"0\",\"notional\":\"0\",\"isolatedWallet\":\"0\",\"updateTime\":0,\"bidNotional\":\"0\",\"askNotional\":\"0\"},{\"symbol\":\"DGBUSDT\",\"initialMargin\":\"0\",\"maintMargin\":\"0\",\"unrealizedProfit\":\"0.00000000\",\"positionInitialMargin\":\"0\",\"openOrderInitialMargin\":\"0\",\"leverage\":\"20\",\"isolated\":false,\"entryPrice\":\"0.0\",\"maxNotional\":\"25000\",\"positionSide\":\"BOTH\",\"positionAmt\":\"0\",\"notional\":\"0\",\"isolatedWallet\":\"0\",\"updateTime\":0,\"bidNotional\":\"0\",\"askNotional\":\"0\"},{\"symbol\":\"SKLUSDT\",\"initialMargin\":\"0\",\"maintMargin\":\"0\",\"unrealizedProfit\":\"0.00000000\",\"positionInitialMargin\":\"0\",\"openOrderInitialMargin\":\"0\",\"leverage\":\"20\",\"isolated\":false,\"entryPrice\":\"0.0\",\"maxNotional\":\"25000\",\"positionSide\":\"BOTH\",\"positionAmt\":\"0\",\"notional\":\"0\",\"isolatedWallet\":\"0\",\"updateTime\":0,\"bidNotional\":\"0\",\"askNotional\":\"0\"},{\"symbol\":\"BTCUSDT_220930\",\"initialMargin\":\"0\",\"maintMargin\":\"0\",\"unrealizedProfit\":\"0.00000000\",\"positionInitialMargin\":\"0\",\"openOrderInitialMargin\":\"0\",\"leverage\":\"25\",\"isolated\":false,\"entryPrice\":\"0.0\",\"maxNotional\":\"375000\",\"positionSide\":\"BOTH\",\"positionAmt\":\"0.000\",\"notional\":\"0\",\"isolatedWallet\":\"0\",\"updateTime\":1658518414311,\"bidNotional\":\"0\",\"askNotional\":\"0\"},{\"symbol\":\"RENUSDT\",\"initialMargin\":\"0\",\"maintMargin\":\"0\",\"unrealizedProfit\":\"0.00000000\",\"positionInitialMargin\":\"0\",\"openOrderInitialMargin\":\"0\",\"leverage\":\"20\",\"isolated\":false,\"entryPrice\":\"0.0\",\"maxNotional\":\"25000\",\"positionSide\":\"BOTH\",\"positionAmt\":\"0\",\"notional\":\"0\",\"isolatedWallet\":\"0\",\"updateTime\":0,\"bidNotional\":\"0\",\"askNotional\":\"0\"},{\"symbol\":\"LPTUSDT\",\"initialMargin\":\"0\",\"maintMargin\":\"0\",\"unrealizedProfit\":\"0.00000000\",\"positionInitialMargin\":\"0\",\"openOrderInitialMargin\":\"0\",\"leverage\":\"20\",\"isolated\":false,\"entryPrice\":\"0.0\",\"maxNotional\":\"25000\",\"positionSide\":\"BOTH\",\"positionAmt\":\"0.0\",\"notional\":\"0\",\"isolatedWallet\":\"0\",\"updateTime\":0,\"bidNotional\":\"0\",\"askNotional\":\"0\"},{\"symbol\":\"JASMYUSDT\",\"initialMargin\":\"0\",\"maintMargin\":\"0\",\"unrealizedProfit\":\"0.00000000\",\"positionInitialMargin\":\"0\",\"openOrderInitialMargin\":\"0\",\"leverage\":\"20\",\"isolated\":false,\"entryPrice\":\"0.0\",\"maxNotional\":\"25000\",\"positionSide\":\"BOTH\",\"positionAmt\":\"0\",\"notional\":\"0\",\"isolatedWallet\":\"0\",\"updateTime\":0,\"bidNotional\":\"0\",\"askNotional\":\"0\"},{\"symbol\":\"TOMOUSDT\",\"initialMargin\":\"0\",\"maintMargin\":\"0\",\"unrealizedProfit\":\"0.00000000\",\"positionInitialMargin\":\"0\",\"openOrderInitialMargin\":\"0\",\"leverage\":\"20\",\"isolated\":false,\"entryPrice\":\"0.0\",\"maxNotional\":\"25000\",\"positionSide\":\"BOTH\",\"positionAmt\":\"0\",\"notional\":\"0\",\"isolatedWallet\":\"0\",\"updateTime\":0,\"bidNotional\":\"0\",\"askNotional\":\"0\"},{\"symbol\":\"MTLUSDT\",\"initialMargin\":\"0\",\"maintMargin\":\"0\",\"unrealizedProfit\":\"0.00000000\",\"positionInitialMargin\":\"0\",\"openOrderInitialMargin\":\"0\",\"leverage\":\"20\",\"isolated\":false,\"entryPrice\":\"0.0\",\"maxNotional\":\"25000\",\"positionSide\":\"BOTH\",\"positionAmt\":\"0\",\"notional\":\"0\",\"isolatedWallet\":\"0\",\"updateTime\":0,\"bidNotional\":\"0\",\"askNotional\":\"0\"},{\"symbol\":\"LTCUSDT\",\"initialMargin\":\"0\",\"maintMargin\":\"0\",\"unrealizedProfit\":\"0.00000000\",\"positionInitialMargin\":\"0\",\"openOrderInitialMargin\":\"0\",\"leverage\":\"3\",\"isolated\":true,\"entryPrice\":\"0.0\",\"maxNotional\":\"10000000\",\"positionSide\":\"BOTH\",\"positionAmt\":\"0.000\",\"notional\":\"0\",\"isolatedWallet\":\"0\",\"updateTime\":0,\"bidNotional\":\"0\",\"askNotional\":\"0\"},{\"symbol\":\"DODOBUSD\",\"initialMargin\":\"0\",\"maintMargin\":\"0\",\"unrealizedProfit\":\"0.00000000\",\"positionInitialMargin\":\"0\",\"openOrderInitialMargin\":\"0\",\"leverage\":\"20\",\"isolated\":false,\"entryPrice\":\"0.0\",\"maxNotional\":\"25000\",\"positionSide\":\"BOTH\",\"positionAmt\":\"0\",\"notional\":\"0\",\"isolatedWallet\":\"0\",\"updateTime\":0,\"bidNotional\":\"0\",\"askNotional\":\"0\"},{\"symbol\":\"EGLDUSDT\",\"initialMargin\":\"0\",\"maintMargin\":\"0\",\"unrealizedProfit\":\"0.00000000\",\"positionInitialMargin\":\"0\",\"openOrderInitialMargin\":\"0\",\"leverage\":\"20\",\"isolated\":false,\"entryPrice\":\"0.0\",\"maxNotional\":\"25000\",\"positionSide\":\"BOTH\",\"positionAmt\":\"0.0\",\"notional\":\"0\",\"isolatedWallet\":\"0\",\"updateTime\":0,\"bidNotional\":\"0\",\"askNotional\":\"0\"},{\"symbol\":\"KSMUSDT\",\"initialMargin\":\"0\",\"maintMargin\":\"0\",\"unrealizedProfit\":\"0.00000000\",\"positionInitialMargin\":\"0\",\"openOrderInitialMargin\":\"0\",\"leverage\":\"20\",\"isolated\":false,\"entryPrice\":\"0.0\",\"maxNotional\":\"25000\",\"positionSide\":\"BOTH\",\"positionAmt\":\"0.0\",\"notional\":\"0\",\"isolatedWallet\":\"0\",\"updateTime\":0,\"bidNotional\":\"0\",\"askNotional\":\"0\"},{\"symbol\":\"WAVESBUSD\",\"initialMargin\":\"0\",\"maintMargin\":\"0\",\"unrealizedProfit\":\"0.00000000\",\"positionInitialMargin\":\"0\",\"openOrderInitialMargin\":\"0\",\"leverage\":\"20\",\"isolated\":false,\"entryPrice\":\"0.0\",\"maxNotional\":\"25000\",\"positionSide\":\"BOTH\",\"positionAmt\":\"0.0\",\"notional\":\"0\",\"isolatedWallet\":\"0\",\"updateTime\":0,\"bidNotional\":\"0\",\"askNotional\":\"0\"},{\"symbol\":\"BNBBUSD\",\"initialMargin\":\"0\",\"maintMargin\":\"0\",\"unrealizedProfit\":\"0.00000000\",\"positionInitialMargin\":\"0\",\"openOrderInitialMargin\":\"0\",\"leverage\":\"20\",\"isolated\":false,\"entryPrice\":\"0.0\",\"maxNotional\":\"100000\",\"positionSide\":\"BOTH\",\"positionAmt\":\"0.00\",\"notional\":\"0\",\"isolatedWallet\":\"0\",\"updateTime\":0,\"bidNotional\":\"0\",\"askNotional\":\"0\"},{\"symbol\":\"ONTUSDT\",\"initialMargin\":\"0\",\"maintMargin\":\"0\",\"unrealizedProfit\":\"0.00000000\",\"positionInitialMargin\":\"0\",\"openOrderInitialMargin\":\"0\",\"leverage\":\"20\",\"isolated\":false,\"entryPrice\":\"0.0\",\"maxNotional\":\"25000\",\"positionSide\":\"BOTH\",\"positionAmt\":\"0.0\",\"notional\":\"0\",\"isolatedWallet\":\"0\",\"updateTime\":0,\"bidNotional\":\"0\",\"askNotional\":\"0\"},{\"symbol\":\"VETUSDT\",\"initialMargin\":\"0\",\"maintMargin\":\"0\",\"unrealizedProfit\":\"0.00000000\",\"positionInitialMargin\":\"0\",\"openOrderInitialMargin\":\"0\",\"leverage\":\"20\",\"isolated\":false,\"entryPrice\":\"0.0\",\"maxNotional\":\"25000\",\"positionSide\":\"BOTH\",\"positionAmt\":\"0\",\"notional\":\"0\",\"isolatedWallet\":\"0\",\"updateTime\":0,\"bidNotional\":\"0\",\"askNotional\":\"0\"},{\"symbol\":\"IMXUSDT\",\"initialMargin\":\"0\",\"maintMargin\":\"0\",\"unrealizedProfit\":\"0.00000000\",\"positionInitialMargin\":\"0\",\"openOrderInitialMargin\":\"0\",\"leverage\":\"20\",\"isolated\":false,\"entryPrice\":\"0.0\",\"maxNotional\":\"25000\",\"positionSide\":\"BOTH\",\"positionAmt\":\"0\",\"notional\":\"0\",\"isolatedWallet\":\"0\",\"updateTime\":0,\"bidNotional\":\"0\",\"askNotional\":\"0\"},{\"symbol\":\"TRBUSDT\",\"initialMargin\":\"0\",\"maintMargin\":\"0\",\"unrealizedProfit\":\"0.00000000\",\"positionInitialMargin\":\"0\",\"openOrderInitialMargin\":\"0\",\"leverage\":\"20\",\"isolated\":false,\"entryPrice\":\"0.0\",\"maxNotional\":\"25000\",\"positionSide\":\"BOTH\",\"positionAmt\":\"0.0\",\"notional\":\"0\",\"isolatedWallet\":\"0\",\"updateTime\":0,\"bidNotional\":\"0\",\"askNotional\":\"0\"},{\"symbol\":\"MANAUSDT\",\"initialMargin\":\"0\",\"maintMargin\":\"0\",\"unrealizedProfit\":\"0.00000000\",\"positionInitialMargin\":\"0\",\"openOrderInitialMargin\":\"0\",\"leverage\":\"3\",\"isolated\":true,\"entryPrice\":\"0.0\",\"maxNotional\":\"1000000\",\"positionSide\":\"BOTH\",\"positionAmt\":\"0\",\"notional\":\"0\",\"isolatedWallet\":\"0\",\"updateTime\":1638400736372,\"bidNotional\":\"0\",\"askNotional\":\"0\"},{\"symbol\":\"FLOWUSDT\",\"initialMargin\":\"0\",\"maintMargin\":\"0\",\"unrealizedProfit\":\"0.00000000\",\"positionInitialMargin\":\"0\",\"openOrderInitialMargin\":\"0\",\"leverage\":\"20\",\"isolated\":false,\"entryPrice\":\"0.0\",\"maxNotional\":\"25000\",\"positionSide\":\"BOTH\",\"positionAmt\":\"0.0\",\"notional\":\"0\",\"isolatedWallet\":\"0\",\"updateTime\":0,\"bidNotional\":\"0\",\"askNotional\":\"0\"},{\"symbol\":\"COTIUSDT\",\"initialMargin\":\"0\",\"maintMargin\":\"0\",\"unrealizedProfit\":\"0.00000000\",\"positionInitialMargin\":\"0\",\"openOrderInitialMargin\":\"0\",\"leverage\":\"20\",\"isolated\":false,\"entryPrice\":\"0.0\",\"maxNotional\":\"25000\",\"positionSide\":\"BOTH\",\"positionAmt\":\"0\",\"notional\":\"0\",\"isolatedWallet\":\"0\",\"updateTime\":0,\"bidNotional\":\"0\",\"askNotional\":\"0\"},{\"symbol\":\"CHRUSDT\",\"initialMargin\":\"0\",\"maintMargin\":\"0\",\"unrealizedProfit\":\"0.00000000\",\"positionInitialMargin\":\"0\",\"openOrderInitialMargin\":\"0\",\"leverage\":\"20\",\"isolated\":false,\"entryPrice\":\"0.0\",\"maxNotional\":\"25000\",\"positionSide\":\"BOTH\",\"positionAmt\":\"0\",\"notional\":\"0\",\"isolatedWallet\":\"0\",\"updateTime\":0,\"bidNotional\":\"0\",\"askNotional\":\"0\"},{\"symbol\":\"BAKEUSDT\",\"initialMargin\":\"0\",\"maintMargin\":\"0\",\"unrealizedProfit\":\"0.00000000\",\"positionInitialMargin\":\"0\",\"openOrderInitialMargin\":\"0\",\"leverage\":\"50\",\"isolated\":false,\"entryPrice\":\"0.0\",\"maxNotional\":\"5000\",\"positionSide\":\"BOTH\",\"positionAmt\":\"0\",\"notional\":\"0\",\"isolatedWallet\":\"0\",\"updateTime\":1653485308830,\"bidNotional\":\"0\",\"askNotional\":\"0\"},{\"symbol\":\"AVAXBUSD\",\"initialMargin\":\"0\",\"maintMargin\":\"0\",\"unrealizedProfit\":\"0.00000000\",\"positionInitialMargin\":\"0\",\"openOrderInitialMargin\":\"0\",\"leverage\":\"20\",\"isolated\":false,\"entryPrice\":\"0.0\",\"maxNotional\":\"25000\",\"positionSide\":\"BOTH\",\"positionAmt\":\"0.0\",\"notional\":\"0\",\"isolatedWallet\":\"0\",\"updateTime\":0,\"bidNotional\":\"0\",\"askNotional\":\"0\"},{\"symbol\":\"GRTUSDT\",\"initialMargin\":\"0\",\"maintMargin\":\"0\",\"unrealizedProfit\":\"0.00000000\",\"positionInitialMargin\":\"0\",\"openOrderInitialMargin\":\"0\",\"leverage\":\"20\",\"isolated\":false,\"entryPrice\":\"0.0\",\"maxNotional\":\"25000\",\"positionSide\":\"BOTH\",\"positionAmt\":\"0\",\"notional\":\"0\",\"isolatedWallet\":\"0\",\"updateTime\":0,\"bidNotional\":\"0\",\"askNotional\":\"0\"},{\"symbol\":\"FLMUSDT\",\"initialMargin\":\"0\",\"maintMargin\":\"0\",\"unrealizedProfit\":\"0.00000000\",\"positionInitialMargin\":\"0\",\"openOrderInitialMargin\":\"0\",\"leverage\":\"20\",\"isolated\":false,\"entryPrice\":\"0.0\",\"maxNotional\":\"25000\",\"positionSide\":\"BOTH\",\"positionAmt\":\"0\",\"notional\":\"0\",\"isolatedWallet\":\"0\",\"updateTime\":0,\"bidNotional\":\"0\",\"askNotional\":\"0\"},{\"symbol\":\"GALUSDT\",\"initialMargin\":\"0\",\"maintMargin\":\"0\",\"unrealizedProfit\":\"0.00000000\",\"positionInitialMargin\":\"0\",\"openOrderInitialMargin\":\"0\",\"leverage\":\"20\",\"isolated\":false,\"entryPrice\":\"0.0\",\"maxNotional\":\"25000\",\"positionSide\":\"BOTH\",\"positionAmt\":\"0\",\"notional\":\"0\",\"isolatedWallet\":\"0\",\"updateTime\":0,\"bidNotional\":\"0\",\"askNotional\":\"0\"},{\"symbol\":\"GALABUSD\",\"initialMargin\":\"0\",\"maintMargin\":\"0\",\"unrealizedProfit\":\"0.00000000\",\"positionInitialMargin\":\"0\",\"openOrderInitialMargin\":\"0\",\"leverage\":\"20\",\"isolated\":false,\"entryPrice\":\"0.0\",\"maxNotional\":\"25000\",\"positionSide\":\"BOTH\",\"positionAmt\":\"0\",\"notional\":\"0\",\"isolatedWallet\":\"0\",\"updateTime\":0,\"bidNotional\":\"0\",\"askNotional\":\"0\"},{\"symbol\":\"MASKUSDT\",\"initialMargin\":\"0\",\"maintMargin\":\"0\",\"unrealizedProfit\":\"0.00000000\",\"positionInitialMargin\":\"0\",\"openOrderInitialMargin\":\"0\",\"leverage\":\"20\",\"isolated\":false,\"entryPrice\":\"0.0\",\"maxNotional\":\"25000\",\"positionSide\":\"BOTH\",\"positionAmt\":\"0\",\"notional\":\"0\",\"isolatedWallet\":\"0\",\"updateTime\":0,\"bidNotional\":\"0\",\"askNotional\":\"0\"},{\"symbol\":\"EOSUSDT\",\"initialMargin\":\"0\",\"maintMargin\":\"0\",\"unrealizedProfit\":\"0.00000000\",\"positionInitialMargin\":\"0\",\"openOrderInitialMargin\":\"0\",\"leverage\":\"3\",\"isolated\":true,\"entryPrice\":\"0.0\",\"maxNotional\":\"10000000\",\"positionSide\":\"BOTH\",\"positionAmt\":\"0.0\",\"notional\":\"0\",\"isolatedWallet\":\"0\",\"updateTime\":1638376997081,\"bidNotional\":\"0\",\"askNotional\":\"0\"},{\"symbol\":\"OGNUSDT\",\"initialMargin\":\"0\",\"maintMargin\":\"0\",\"unrealizedProfit\":\"0.00000000\",\"positionInitialMargin\":\"0\",\"openOrderInitialMargin\":\"0\",\"leverage\":\"20\",\"isolated\":false,\"entryPrice\":\"0.0\",\"maxNotional\":\"25000\",\"positionSide\":\"BOTH\",\"positionAmt\":\"0\",\"notional\":\"0\",\"isolatedWallet\":\"0\",\"updateTime\":0,\"bidNotional\":\"0\",\"askNotional\":\"0\"},{\"symbol\":\"SCUSDT\",\"initialMargin\":\"0\",\"maintMargin\":\"0\",\"unrealizedProfit\":\"0.00000000\",\"positionInitialMargin\":\"0\",\"openOrderInitialMargin\":\"0\",\"leverage\":\"20\",\"isolated\":false,\"entryPrice\":\"0.0\",\"maxNotional\":\"25000\",\"positionSide\":\"BOTH\",\"positionAmt\":\"0\",\"notional\":\"0\",\"isolatedWallet\":\"0\",\"updateTime\":0,\"bidNotional\":\"0\",\"askNotional\":\"0\"},{\"symbol\":\"GALBUSD\",\"initialMargin\":\"0\",\"maintMargin\":\"0\",\"unrealizedProfit\":\"0.00000000\",\"positionInitialMargin\":\"0\",\"openOrderInitialMargin\":\"0\",\"leverage\":\"20\",\"isolated\":false,\"entryPrice\":\"0.0\",\"maxNotional\":\"25000\",\"positionSide\":\"BOTH\",\"positionAmt\":\"0\",\"notional\":\"0\",\"isolatedWallet\":\"0\",\"updateTime\":0,\"bidNotional\":\"0\",\"askNotional\":\"0\"},{\"symbol\":\"BALUSDT\",\"initialMargin\":\"0\",\"maintMargin\":\"0\",\"unrealizedProfit\":\"0.00000000\",\"positionInitialMargin\":\"0\",\"openOrderInitialMargin\":\"0\",\"leverage\":\"20\",\"isolated\":false,\"entryPrice\":\"0.0\",\"maxNotional\":\"25000\",\"positionSide\":\"BOTH\",\"positionAmt\":\"0.0\",\"notional\":\"0\",\"isolatedWallet\":\"0\",\"updateTime\":0,\"bidNotional\":\"0\",\"askNotional\":\"0\"},{\"symbol\":\"STMXUSDT\",\"initialMargin\":\"0\",\"maintMargin\":\"0\",\"unrealizedProfit\":\"0.00000000\",\"positionInitialMargin\":\"0\",\"openOrderInitialMargin\":\"0\",\"leverage\":\"20\",\"isolated\":false,\"entryPrice\":\"0.0\",\"maxNotional\":\"25000\",\"positionSide\":\"BOTH\",\"positionAmt\":\"0\",\"notional\":\"0\",\"isolatedWallet\":\"0\",\"updateTime\":0,\"bidNotional\":\"0\",\"askNotional\":\"0\"},{\"symbol\":\"DENTUSDT\",\"initialMargin\":\"0\",\"maintMargin\":\"0\",\"unrealizedProfit\":\"0.00000000\",\"positionInitialMargin\":\"0\",\"openOrderInitialMargin\":\"0\",\"leverage\":\"20\",\"isolated\":false,\"entryPrice\":\"0.0\",\"maxNotional\":\"25000\",\"positionSide\":\"BOTH\",\"positionAmt\":\"0\",\"notional\":\"0\",\"isolatedWallet\":\"0\",\"updateTime\":0,\"bidNotional\":\"0\",\"askNotional\":\"0\"},{\"symbol\":\"KNCUSDT\",\"initialMargin\":\"0\",\"maintMargin\":\"0\",\"unrealizedProfit\":\"0.00000000\",\"positionInitialMargin\":\"0\",\"openOrderInitialMargin\":\"0\",\"leverage\":\"20\",\"isolated\":false,\"entryPrice\":\"0.0\",\"maxNotional\":\"25000\",\"positionSide\":\"BOTH\",\"positionAmt\":\"0\",\"notional\":\"0\",\"isolatedWallet\":\"0\",\"updateTime\":0,\"bidNotional\":\"0\",\"askNotional\":\"0\"},{\"symbol\":\"SRMUSDT\",\"initialMargin\":\"0\",\"maintMargin\":\"0\",\"unrealizedProfit\":\"0.00000000\",\"positionInitialMargin\":\"0\",\"openOrderInitialMargin\":\"0\",\"leverage\":\"20\",\"isolated\":false,\"entryPrice\":\"0.0\",\"maxNotional\":\"25000\",\"positionSide\":\"BOTH\",\"positionAmt\":\"0\",\"notional\":\"0\",\"isolatedWallet\":\"0\",\"updateTime\":0,\"bidNotional\":\"0\",\"askNotional\":\"0\"},{\"symbol\":\"ENJUSDT\",\"initialMargin\":\"0\",\"maintMargin\":\"0\",\"unrealizedProfit\":\"0.00000000\",\"positionInitialMargin\":\"0\",\"openOrderInitialMargin\":\"0\",\"leverage\":\"20\",\"isolated\":false,\"entryPrice\":\"0.0\",\"maxNotional\":\"150000\",\"positionSide\":\"BOTH\",\"positionAmt\":\"0\",\"notional\":\"0\",\"isolatedWallet\":\"0\",\"updateTime\":0,\"bidNotional\":\"0\",\"askNotional\":\"0\"},{\"symbol\":\"MATICBUSD\",\"initialMargin\":\"0\",\"maintMargin\":\"0\",\"unrealizedProfit\":\"0.00000000\",\"positionInitialMargin\":\"0\",\"openOrderInitialMargin\":\"0\",\"leverage\":\"20\",\"isolated\":false,\"entryPrice\":\"0.0\",\"maxNotional\":\"25000\",\"positionSide\":\"BOTH\",\"positionAmt\":\"0\",\"notional\":\"0\",\"isolatedWallet\":\"0\",\"updateTime\":0,\"bidNotional\":\"0\",\"askNotional\":\"0\"},{\"symbol\":\"C98USDT\",\"initialMargin\":\"0\",\"maintMargin\":\"0\",\"unrealizedProfit\":\"0.00000000\",\"positionInitialMargin\":\"0\",\"openOrderInitialMargin\":\"0\",\"leverage\":\"20\",\"isolated\":false,\"entryPrice\":\"0.0\",\"maxNotional\":\"25000\",\"positionSide\":\"BOTH\",\"positionAmt\":\"0\",\"notional\":\"0\",\"isolatedWallet\":\"0\",\"updateTime\":0,\"bidNotional\":\"0\",\"askNotional\":\"0\"},{\"symbol\":\"ZENUSDT\",\"initialMargin\":\"0\",\"maintMargin\":\"0\",\"unrealizedProfit\":\"0.00000000\",\"positionInitialMargin\":\"0\",\"openOrderInitialMargin\":\"0\",\"leverage\":\"20\",\"isolated\":false,\"entryPrice\":\"0.0\",\"maxNotional\":\"25000\",\"positionSide\":\"BOTH\",\"positionAmt\":\"0.0\",\"notional\":\"0\",\"isolatedWallet\":\"0\",\"updateTime\":0,\"bidNotional\":\"0\",\"askNotional\":\"0\"},{\"symbol\":\"ATOMUSDT\",\"initialMargin\":\"0\",\"maintMargin\":\"0\",\"unrealizedProfit\":\"0.00000000\",\"positionInitialMargin\":\"0\",\"openOrderInitialMargin\":\"0\",\"leverage\":\"20\",\"isolated\":false,\"entryPrice\":\"0.0\",\"maxNotional\":\"25000\",\"positionSide\":\"BOTH\",\"positionAmt\":\"0.00\",\"notional\":\"0\",\"isolatedWallet\":\"0\",\"updateTime\":0,\"bidNotional\":\"0\",\"askNotional\":\"0\"},{\"symbol\":\"NEARUSDT\",\"initialMargin\":\"0\",\"maintMargin\":\"0\",\"unrealizedProfit\":\"0.00000000\",\"positionInitialMargin\":\"0\",\"openOrderInitialMargin\":\"0\",\"leverage\":\"20\",\"isolated\":false,\"entryPrice\":\"0.0\",\"maxNotional\":\"150000\",\"positionSide\":\"BOTH\",\"positionAmt\":\"0\",\"notional\":\"0\",\"isolatedWallet\":\"0\",\"updateTime\":0,\"bidNotional\":\"0\",\"askNotional\":\"0\"},{\"symbol\":\"SOLBUSD\",\"initialMargin\":\"0\",\"maintMargin\":\"0\",\"unrealizedProfit\":\"0.00000000\",\"positionInitialMargin\":\"0\",\"openOrderInitialMargin\":\"0\",\"leverage\":\"20\",\"isolated\":false,\"entryPrice\":\"0.0\",\"maxNotional\":\"100000\",\"positionSide\":\"BOTH\",\"positionAmt\":\"0\",\"notional\":\"0\",\"isolatedWallet\":\"0\",\"updateTime\":0,\"bidNotional\":\"0\",\"askNotional\":\"0\"},{\"symbol\":\"ENSUSDT\",\"initialMargin\":\"0\",\"maintMargin\":\"0\",\"unrealizedProfit\":\"0.00000000\",\"positionInitialMargin\":\"0\",\"openOrderInitialMargin\":\"0\",\"leverage\":\"20\",\"isolated\":false,\"entryPrice\":\"0.0\",\"maxNotional\":\"25000\",\"positionSide\":\"BOTH\",\"positionAmt\":\"0.0\",\"notional\":\"0\",\"isolatedWallet\":\"0\",\"updateTime\":0,\"bidNotional\":\"0\",\"askNotional\":\"0\"},{\"symbol\":\"FILBUSD\",\"initialMargin\":\"0\",\"maintMargin\":\"0\",\"unrealizedProfit\":\"0.00000000\",\"positionInitialMargin\":\"0\",\"openOrderInitialMargin\":\"0\",\"leverage\":\"20\",\"isolated\":false,\"entryPrice\":\"0.0\",\"maxNotional\":\"25000\",\"positionSide\":\"BOTH\",\"positionAmt\":\"0.0\",\"notional\":\"0\",\"isolatedWallet\":\"0\",\"updateTime\":0,\"bidNotional\":\"0\",\"askNotional\":\"0\"},{\"symbol\":\"BCHUSDT\",\"initialMargin\":\"0\",\"maintMargin\":\"0\",\"unrealizedProfit\":\"0.00000000\",\"positionInitialMargin\":\"0\",\"openOrderInitialMargin\":\"0\",\"leverage\":\"3\",\"isolated\":true,\"entryPrice\":\"0.0\",\"maxNotional\":\"10000000\",\"positionSide\":\"BOTH\",\"positionAmt\":\"0.000\",\"notional\":\"0\",\"isolatedWallet\":\"0\",\"updateTime\":1638373241266,\"bidNotional\":\"0\",\"askNotional\":\"0\"},{\"symbol\":\"ATAUSDT\",\"initialMargin\":\"0\",\"maintMargin\":\"0\",\"unrealizedProfit\":\"0.00000000\",\"positionInitialMargin\":\"0\",\"openOrderInitialMargin\":\"0\",\"leverage\":\"25\",\"isolated\":false,\"entryPrice\":\"0.0\",\"maxNotional\":\"5000\",\"positionSide\":\"BOTH\",\"positionAmt\":\"0\",\"notional\":\"0\",\"isolatedWallet\":\"0\",\"updateTime\":1653491919372,\"bidNotional\":\"0\",\"askNotional\":\"0\"},{\"symbol\":\"IOSTUSDT\",\"initialMargin\":\"0\",\"maintMargin\":\"0\",\"unrealizedProfit\":\"0.00000000\",\"positionInitialMargin\":\"0\",\"openOrderInitialMargin\":\"0\",\"leverage\":\"20\",\"isolated\":false,\"entryPrice\":\"0.0\",\"maxNotional\":\"25000\",\"positionSide\":\"BOTH\",\"positionAmt\":\"0\",\"notional\":\"0\",\"isolatedWallet\":\"0\",\"updateTime\":0,\"bidNotional\":\"0\",\"askNotional\":\"0\"},{\"symbol\":\"HBARUSDT\",\"initialMargin\":\"0\",\"maintMargin\":\"0\",\"unrealizedProfit\":\"0.00000000\",\"positionInitialMargin\":\"0\",\"openOrderInitialMargin\":\"0\",\"leverage\":\"20\",\"isolated\":false,\"entryPrice\":\"0.0\",\"maxNotional\":\"25000\",\"positionSide\":\"BOTH\",\"positionAmt\":\"0\",\"notional\":\"0\",\"isolatedWallet\":\"0\",\"updateTime\":0,\"bidNotional\":\"0\",\"askNotional\":\"0\"},{\"symbol\":\"LUNA2BUSD\",\"initialMargin\":\"0\",\"maintMargin\":\"0\",\"unrealizedProfit\":\"0.00000000\",\"positionInitialMargin\":\"0\",\"openOrderInitialMargin\":\"0\",\"leverage\":\"20\",\"isolated\":false,\"entryPrice\":\"0.0\",\"maxNotional\":\"25000\",\"positionSide\":\"BOTH\",\"positionAmt\":\"0\",\"notional\":\"0\",\"isolatedWallet\":\"0\",\"updateTime\":0,\"bidNotional\":\"0\",\"askNotional\":\"0\"},{\"symbol\":\"LTCBUSD\",\"initialMargin\":\"0\",\"maintMargin\":\"0\",\"unrealizedProfit\":\"0.00000000\",\"positionInitialMargin\":\"0\",\"openOrderInitialMargin\":\"0\",\"leverage\":\"20\",\"isolated\":false,\"entryPrice\":\"0.0\",\"maxNotional\":\"25000\",\"positionSide\":\"BOTH\",\"positionAmt\":\"0.00\",\"notional\":\"0\",\"isolatedWallet\":\"0\",\"updateTime\":0,\"bidNotional\":\"0\",\"askNotional\":\"0\"},{\"symbol\":\"ZECUSDT\",\"initialMargin\":\"0\",\"maintMargin\":\"0\",\"unrealizedProfit\":\"0.00000000\",\"positionInitialMargin\":\"0\",\"openOrderInitialMargin\":\"0\",\"leverage\":\"20\",\"isolated\":false,\"entryPrice\":\"0.0\",\"maxNotional\":\"150000\",\"positionSide\":\"BOTH\",\"positionAmt\":\"0.000\",\"notional\":\"0\",\"isolatedWallet\":\"0\",\"updateTime\":0,\"bidNotional\":\"0\",\"askNotional\":\"0\"},{\"symbol\":\"1000SHIBUSDT\",\"initialMargin\":\"0\",\"maintMargin\":\"0\",\"unrealizedProfit\":\"0.00000000\",\"positionInitialMargin\":\"0\",\"openOrderInitialMargin\":\"0\",\"leverage\":\"3\",\"isolated\":true,\"entryPrice\":\"0.0\",\"maxNotional\":\"1000000\",\"positionSide\":\"BOTH\",\"positionAmt\":\"0\",\"notional\":\"0\",\"isolatedWallet\":\"0\",\"updateTime\":0,\"bidNotional\":\"0\",\"askNotional\":\"0\"},{\"symbol\":\"TLMBUSD\",\"initialMargin\":\"0\",\"maintMargin\":\"0\",\"unrealizedProfit\":\"0.00000000\",\"positionInitialMargin\":\"0\",\"openOrderInitialMargin\":\"0\",\"leverage\":\"20\",\"isolated\":false,\"entryPrice\":\"0.0\",\"maxNotional\":\"25000\",\"positionSide\":\"BOTH\",\"positionAmt\":\"0\",\"notional\":\"0\",\"isolatedWallet\":\"0\",\"updateTime\":0,\"bidNotional\":\"0\",\"askNotional\":\"0\"},{\"symbol\":\"TLMUSDT\",\"initialMargin\":\"0\",\"maintMargin\":\"0\",\"unrealizedProfit\":\"0.00000000\",\"positionInitialMargin\":\"0\",\"openOrderInitialMargin\":\"0\",\"leverage\":\"20\",\"isolated\":false,\"entryPrice\":\"0.0\",\"maxNotional\":\"25000\",\"positionSide\":\"BOTH\",\"positionAmt\":\"0\",\"notional\":\"0\",\"isolatedWallet\":\"0\",\"updateTime\":0,\"bidNotional\":\"0\",\"askNotional\":\"0\"},{\"symbol\":\"ANTUSDT\",\"initialMargin\":\"0\",\"maintMargin\":\"0\",\"unrealizedProfit\":\"0.00000000\",\"positionInitialMargin\":\"0\",\"openOrderInitialMargin\":\"0\",\"leverage\":\"20\",\"isolated\":false,\"entryPrice\":\"0.0\",\"maxNotional\":\"25000\",\"positionSide\":\"BOTH\",\"positionAmt\":\"0.0\",\"notional\":\"0\",\"isolatedWallet\":\"0\",\"updateTime\":0,\"bidNotional\":\"0\",\"askNotional\":\"0\"},{\"symbol\":\"ETHBUSD\",\"initialMargin\":\"0\",\"maintMargin\":\"0\",\"unrealizedProfit\":\"0.00000000\",\"positionInitialMargin\":\"0\",\"openOrderInitialMargin\":\"0\",\"leverage\":\"20\",\"isolated\":false,\"entryPrice\":\"0.0\",\"maxNotional\":\"500000\",\"positionSide\":\"BOTH\",\"positionAmt\":\"0.000\",\"notional\":\"0\",\"isolatedWallet\":\"0\",\"updateTime\":0,\"bidNotional\":\"0\",\"askNotional\":\"0\"},{\"symbol\":\"GALAUSDT\",\"initialMargin\":\"0\",\"maintMargin\":\"0\",\"unrealizedProfit\":\"0.00000000\",\"positionInitialMargin\":\"0\",\"openOrderInitialMargin\":\"0\",\"leverage\":\"10\",\"isolated\":false,\"entryPrice\":\"0.0\",\"maxNotional\":\"100000\",\"positionSide\":\"BOTH\",\"positionAmt\":\"0\",\"notional\":\"0\",\"isolatedWallet\":\"0\",\"updateTime\":0,\"bidNotional\":\"0\",\"askNotional\":\"0\"},{\"symbol\":\"AAVEUSDT\",\"initialMargin\":\"0\",\"maintMargin\":\"0\",\"unrealizedProfit\":\"0.00000000\",\"positionInitialMargin\":\"0\",\"openOrderInitialMargin\":\"0\",\"leverage\":\"20\",\"isolated\":false,\"entryPrice\":\"0.0\",\"maxNotional\":\"25000\",\"positionSide\":\"BOTH\",\"positionAmt\":\"0.0\",\"notional\":\"0\",\"isolatedWallet\":\"0\",\"updateTime\":0,\"bidNotional\":\"0\",\"askNotional\":\"0\"},{\"symbol\":\"GTCUSDT\",\"initialMargin\":\"0\",\"maintMargin\":\"0\",\"unrealizedProfit\":\"0.00000000\",\"positionInitialMargin\":\"0\",\"openOrderInitialMargin\":\"0\",\"leverage\":\"20\",\"isolated\":false,\"entryPrice\":\"0.0\",\"maxNotional\":\"25000\",\"positionSide\":\"BOTH\",\"positionAmt\":\"0.0\",\"notional\":\"0\",\"isolatedWallet\":\"0\",\"updateTime\":0,\"bidNotional\":\"0\",\"askNotional\":\"0\"},{\"symbol\":\"ALGOUSDT\",\"initialMargin\":\"0\",\"maintMargin\":\"0\",\"unrealizedProfit\":\"0.00000000\",\"positionInitialMargin\":\"0\",\"openOrderInitialMargin\":\"0\",\"leverage\":\"3\",\"isolated\":false,\"entryPrice\":\"0.0\",\"maxNotional\":\"250000\",\"positionSide\":\"BOTH\",\"positionAmt\":\"0.0\",\"notional\":\"0\",\"isolatedWallet\":\"0\",\"updateTime\":1638373624088,\"bidNotional\":\"0\",\"askNotional\":\"0\"},{\"symbol\":\"ICPUSDT\",\"initialMargin\":\"0\",\"maintMargin\":\"0\",\"unrealizedProfit\":\"0.00000000\",\"positionInitialMargin\":\"0\",\"openOrderInitialMargin\":\"0\",\"leverage\":\"20\",\"isolated\":false,\"entryPrice\":\"0.0\",\"maxNotional\":\"25000\",\"positionSide\":\"BOTH\",\"positionAmt\":\"0.00\",\"notional\":\"0\",\"isolatedWallet\":\"0\",\"updateTime\":0,\"bidNotional\":\"0\",\"askNotional\":\"0\"},{\"symbol\":\"LRCUSDT\",\"initialMargin\":\"0\",\"maintMargin\":\"0\",\"unrealizedProfit\":\"0.00000000\",\"positionInitialMargin\":\"0\",\"openOrderInitialMargin\":\"0\",\"leverage\":\"3\",\"isolated\":true,\"entryPrice\":\"0.0\",\"maxNotional\":\"250000\",\"positionSide\":\"BOTH\",\"positionAmt\":\"0\",\"notional\":\"0\",\"isolatedWallet\":\"0\",\"updateTime\":1638376754291,\"bidNotional\":\"0\",\"askNotional\":\"0\"},{\"symbol\":\"AVAXUSDT\",\"initialMargin\":\"0\",\"maintMargin\":\"0\",\"unrealizedProfit\":\"0.00000000\",\"positionInitialMargin\":\"0\",\"openOrderInitialMargin\":\"0\",\"leverage\":\"3\",\"isolated\":true,\"entryPrice\":\"0.0\",\"maxNotional\":\"5000000\",\"positionSide\":\"BOTH\",\"positionAmt\":\"0\",\"notional\":\"0\",\"isolatedWallet\":\"0\",\"updateTime\":1636890309205,\"bidNotional\":\"0\",\"askNotional\":\"0\"},{\"symbol\":\"ARPAUSDT\",\"initialMargin\":\"0\",\"maintMargin\":\"0\",\"unrealizedProfit\":\"0.00000000\",\"positionInitialMargin\":\"0\",\"openOrderInitialMargin\":\"0\",\"leverage\":\"20\",\"isolated\":false,\"entryPrice\":\"0.0\",\"maxNotional\":\"25000\",\"positionSide\":\"BOTH\",\"positionAmt\":\"0\",\"notional\":\"0\",\"isolatedWallet\":\"0\",\"updateTime\":0,\"bidNotional\":\"0\",\"askNotional\":\"0\"},{\"symbol\":\"CELOUSDT\",\"initialMargin\":\"0\",\"maintMargin\":\"0\",\"unrealizedProfit\":\"0.00000000\",\"positionInitialMargin\":\"0\",\"openOrderInitialMargin\":\"0\",\"leverage\":\"20\",\"isolated\":false,\"entryPrice\":\"0.0\",\"maxNotional\":\"25000\",\"positionSide\":\"BOTH\",\"positionAmt\":\"0.0\",\"notional\":\"0\",\"isolatedWallet\":\"0\",\"updateTime\":0,\"bidNotional\":\"0\",\"askNotional\":\"0\"},{\"symbol\":\"ROSEUSDT\",\"initialMargin\":\"0\",\"maintMargin\":\"0\",\"unrealizedProfit\":\"0.00000000\",\"positionInitialMargin\":\"0\",\"openOrderInitialMargin\":\"0\",\"leverage\":\"20\",\"isolated\":false,\"entryPrice\":\"0.0\",\"maxNotional\":\"25000\",\"positionSide\":\"BOTH\",\"positionAmt\":\"0\",\"notional\":\"0\",\"isolatedWallet\":\"0\",\"updateTime\":0,\"bidNotional\":\"0\",\"askNotional\":\"0\"},{\"symbol\":\"MATICUSDT\",\"initialMargin\":\"0\",\"maintMargin\":\"0\",\"unrealizedProfit\":\"0.00000000\",\"positionInitialMargin\":\"0\",\"openOrderInitialMargin\":\"0\",\"leverage\":\"20\",\"isolated\":false,\"entryPrice\":\"0.0\",\"maxNotional\":\"150000\",\"positionSide\":\"BOTH\",\"positionAmt\":\"0\",\"notional\":\"0\",\"isolatedWallet\":\"0\",\"updateTime\":0,\"bidNotional\":\"0\",\"askNotional\":\"0\"},{\"symbol\":\"1INCHUSDT\",\"initialMargin\":\"0\",\"maintMargin\":\"0\",\"unrealizedProfit\":\"0.00000000\",\"positionInitialMargin\":\"0\",\"openOrderInitialMargin\":\"0\",\"leverage\":\"20\",\"isolated\":false,\"entryPrice\":\"0.0\",\"maxNotional\":\"25000\",\"positionSide\":\"BOTH\",\"positionAmt\":\"0\",\"notional\":\"0\",\"isolatedWallet\":\"0\",\"updateTime\":0,\"bidNotional\":\"0\",\"askNotional\":\"0\"},{\"symbol\":\"MKRUSDT\",\"initialMargin\":\"0\",\"maintMargin\":\"0\",\"unrealizedProfit\":\"0.00000000\",\"positionInitialMargin\":\"0\",\"openOrderInitialMargin\":\"0\",\"leverage\":\"20\",\"isolated\":false,\"entryPrice\":\"0.0\",\"maxNotional\":\"25000\",\"positionSide\":\"BOTH\",\"positionAmt\":\"0.000\",\"notional\":\"0\",\"isolatedWallet\":\"0\",\"updateTime\":0,\"bidNotional\":\"0\",\"askNotional\":\"0\"},{\"symbol\":\"PEOPLEUSDT\",\"initialMargin\":\"0\",\"maintMargin\":\"0\",\"unrealizedProfit\":\"0.00000000\",\"positionInitialMargin\":\"0\",\"openOrderInitialMargin\":\"0\",\"leverage\":\"20\",\"isolated\":false,\"entryPrice\":\"0.0\",\"maxNotional\":\"25000\",\"positionSide\":\"BOTH\",\"positionAmt\":\"0\",\"notional\":\"0\",\"isolatedWallet\":\"0\",\"updateTime\":0,\"bidNotional\":\"0\",\"askNotional\":\"0\"},{\"symbol\":\"ANCBUSD\",\"initialMargin\":\"0\",\"maintMargin\":\"0\",\"unrealizedProfit\":\"0.00000000\",\"positionInitialMargin\":\"0\",\"openOrderInitialMargin\":\"0\",\"leverage\":\"20\",\"isolated\":false,\"entryPrice\":\"0.0\",\"maxNotional\":\"25000\",\"positionSide\":\"BOTH\",\"positionAmt\":\"0\",\"notional\":\"0\",\"isolatedWallet\":\"0\",\"updateTime\":0,\"bidNotional\":\"0\",\"askNotional\":\"0\"},{\"symbol\":\"THETAUSDT\",\"initialMargin\":\"0\",\"maintMargin\":\"0\",\"unrealizedProfit\":\"0.00000000\",\"positionInitialMargin\":\"0\",\"openOrderInitialMargin\":\"0\",\"leverage\":\"20\",\"isolated\":false,\"entryPrice\":\"0.0\",\"maxNotional\":\"250000\",\"positionSide\":\"BOTH\",\"positionAmt\":\"0.0\",\"notional\":\"0\",\"isolatedWallet\":\"0\",\"updateTime\":0,\"bidNotional\":\"0\",\"askNotional\":\"0\"},{\"symbol\":\"UNIUSDT\",\"initialMargin\":\"0\",\"maintMargin\":\"0\",\"unrealizedProfit\":\"0.00000000\",\"positionInitialMargin\":\"0\",\"openOrderInitialMargin\":\"0\",\"leverage\":\"20\",\"isolated\":false,\"entryPrice\":\"0.0\",\"maxNotional\":\"25000\",\"positionSide\":\"BOTH\",\"positionAmt\":\"0\",\"notional\":\"0\",\"isolatedWallet\":\"0\",\"updateTime\":0,\"bidNotional\":\"0\",\"askNotional\":\"0\"},{\"symbol\":\"LINAUSDT\",\"initialMargin\":\"0\",\"maintMargin\":\"0\",\"unrealizedProfit\":\"0.00000000\",\"positionInitialMargin\":\"0\",\"openOrderInitialMargin\":\"0\",\"leverage\":\"20\",\"isolated\":false,\"entryPrice\":\"0.0\",\"maxNotional\":\"25000\",\"positionSide\":\"BOTH\",\"positionAmt\":\"0\",\"notional\":\"0\",\"isolatedWallet\":\"0\",\"updateTime\":0,\"bidNotional\":\"0\",\"askNotional\":\"0\"},{\"symbol\":\"ARUSDT\",\"initialMargin\":\"0\",\"maintMargin\":\"0\",\"unrealizedProfit\":\"0.00000000\",\"positionInitialMargin\":\"0\",\"openOrderInitialMargin\":\"0\",\"leverage\":\"20\",\"isolated\":false,\"entryPrice\":\"0.0\",\"maxNotional\":\"25000\",\"positionSide\":\"BOTH\",\"positionAmt\":\"0.0\",\"notional\":\"0\",\"isolatedWallet\":\"0\",\"updateTime\":0,\"bidNotional\":\"0\",\"askNotional\":\"0\"},{\"symbol\":\"RVNUSDT\",\"initialMargin\":\"0\",\"maintMargin\":\"0\",\"unrealizedProfit\":\"0.00000000\",\"positionInitialMargin\":\"0\",\"openOrderInitialMargin\":\"0\",\"leverage\":\"20\",\"isolated\":false,\"entryPrice\":\"0.0\",\"maxNotional\":\"25000\",\"positionSide\":\"BOTH\",\"positionAmt\":\"0\",\"notional\":\"0\",\"isolatedWallet\":\"0\",\"updateTime\":0,\"bidNotional\":\"0\",\"askNotional\":\"0\"},{\"symbol\":\"FILUSDT\",\"initialMargin\":\"0\",\"maintMargin\":\"0\",\"unrealizedProfit\":\"0.00000000\",\"positionInitialMargin\":\"0\",\"openOrderInitialMargin\":\"0\",\"leverage\":\"20\",\"isolated\":false,\"entryPrice\":\"0.0\",\"maxNotional\":\"250000\",\"positionSide\":\"BOTH\",\"positionAmt\":\"0.0\",\"notional\":\"0\",\"isolatedWallet\":\"0\",\"updateTime\":0,\"bidNotional\":\"0\",\"askNotional\":\"0\"},{\"symbol\":\"NKNUSDT\",\"initialMargin\":\"0\",\"maintMargin\":\"0\",\"unrealizedProfit\":\"0.00000000\",\"positionInitialMargin\":\"0\",\"openOrderInitialMargin\":\"0\",\"leverage\":\"20\",\"isolated\":false,\"entryPrice\":\"0.0\",\"maxNotional\":\"25000\",\"positionSide\":\"BOTH\",\"positionAmt\":\"0\",\"notional\":\"0\",\"isolatedWallet\":\"0\",\"updateTime\":0,\"bidNotional\":\"0\",\"askNotional\":\"0\"},{\"symbol\":\"KLAYUSDT\",\"initialMargin\":\"0\",\"maintMargin\":\"0\",\"unrealizedProfit\":\"0.00000000\",\"positionInitialMargin\":\"0\",\"openOrderInitialMargin\":\"0\",\"leverage\":\"20\",\"isolated\":false,\"entryPrice\":\"0.0\",\"maxNotional\":\"25000\",\"positionSide\":\"BOTH\",\"positionAmt\":\"0.0\",\"notional\":\"0\",\"isolatedWallet\":\"0\",\"updateTime\":0,\"bidNotional\":\"0\",\"askNotional\":\"0\"},{\"symbol\":\"DEFIUSDT\",\"initialMargin\":\"0\",\"maintMargin\":\"0\",\"unrealizedProfit\":\"0.00000000\",\"positionInitialMargin\":\"0\",\"openOrderInitialMargin\":\"0\",\"leverage\":\"20\",\"isolated\":false,\"entryPrice\":\"0.0\",\"maxNotional\":\"25000\",\"positionSide\":\"BOTH\",\"positionAmt\":\"0.000\",\"notional\":\"0\",\"isolatedWallet\":\"0\",\"updateTime\":0,\"bidNotional\":\"0\",\"askNotional\":\"0\"},{\"symbol\":\"COMPUSDT\",\"initialMargin\":\"0\",\"maintMargin\":\"0\",\"unrealizedProfit\":\"0.00000000\",\"positionInitialMargin\":\"0\",\"openOrderInitialMargin\":\"0\",\"leverage\":\"20\",\"isolated\":false,\"entryPrice\":\"0.0\",\"maxNotional\":\"25000\",\"positionSide\":\"BOTH\",\"positionAmt\":\"0.000\",\"notional\":\"0\",\"isolatedWallet\":\"0\",\"updateTime\":0,\"bidNotional\":\"0\",\"askNotional\":\"0\"},{\"symbol\":\"BTCDOMUSDT\",\"initialMargin\":\"0\",\"maintMargin\":\"0\",\"unrealizedProfit\":\"0.00000000\",\"positionInitialMargin\":\"0\",\"openOrderInitialMargin\":\"0\",\"leverage\":\"20\",\"isolated\":false,\"entryPrice\":\"0.0\",\"maxNotional\":\"25000\",\"positionSide\":\"BOTH\",\"positionAmt\":\"0.000\",\"notional\":\"0\",\"isolatedWallet\":\"0\",\"updateTime\":0,\"bidNotional\":\"0\",\"askNotional\":\"0\"},{\"symbol\":\"SOLUSDT\",\"initialMargin\":\"0\",\"maintMargin\":\"0\",\"unrealizedProfit\":\"0.00000000\",\"positionInitialMargin\":\"0\",\"openOrderInitialMargin\":\"0\",\"leverage\":\"3\",\"isolated\":true,\"entryPrice\":\"0.0\",\"maxNotional\":\"5000000\",\"positionSide\":\"BOTH\",\"positionAmt\":\"0\",\"notional\":\"0\",\"isolatedWallet\":\"0\",\"updateTime\":0,\"bidNotional\":\"0\",\"askNotional\":\"0\"},{\"symbol\":\"BTCUSDT\",\"initialMargin\":\"0\",\"maintMargin\":\"0\",\"unrealizedProfit\":\"0.00000000\",\"positionInitialMargin\":\"0\",\"openOrderInitialMargin\":\"0\",\"leverage\":\"20\",\"isolated\":true,\"entryPrice\":\"0.0\",\"maxNotional\":\"10000000\",\"positionSide\":\"BOTH\",\"positionAmt\":\"0.000\",\"notional\":\"0\",\"isolatedWallet\":\"0\",\"updateTime\":1655799488436,\"bidNotional\":\"0\",\"askNotional\":\"0\"},{\"symbol\":\"OMGUSDT\",\"initialMargin\":\"0\",\"maintMargin\":\"0\",\"unrealizedProfit\":\"0.00000000\",\"positionInitialMargin\":\"0\",\"openOrderInitialMargin\":\"0\",\"leverage\":\"20\",\"isolated\":false,\"entryPrice\":\"0.0\",\"maxNotional\":\"25000\",\"positionSide\":\"BOTH\",\"positionAmt\":\"0.0\",\"notional\":\"0\",\"isolatedWallet\":\"0\",\"updateTime\":0,\"bidNotional\":\"0\",\"askNotional\":\"0\"},{\"symbol\":\"ICXUSDT\",\"initialMargin\":\"0\",\"maintMargin\":\"0\",\"unrealizedProfit\":\"0.00000000\",\"positionInitialMargin\":\"0\",\"openOrderInitialMargin\":\"0\",\"leverage\":\"20\",\"isolated\":false,\"entryPrice\":\"0.0\",\"maxNotional\":\"25000\",\"positionSide\":\"BOTH\",\"positionAmt\":\"0\",\"notional\":\"0\",\"isolatedWallet\":\"0\",\"updateTime\":0,\"bidNotional\":\"0\",\"askNotional\":\"0\"},{\"symbol\":\"ICPBUSD\",\"initialMargin\":\"0\",\"maintMargin\":\"0\",\"unrealizedProfit\":\"0.00000000\",\"positionInitialMargin\":\"0\",\"openOrderInitialMargin\":\"0\",\"leverage\":\"20\",\"isolated\":false,\"entryPrice\":\"0.0\",\"maxNotional\":\"25000\",\"positionSide\":\"BOTH\",\"positionAmt\":\"0.0\",\"notional\":\"0\",\"isolatedWallet\":\"0\",\"updateTime\":0,\"bidNotional\":\"0\",\"askNotional\":\"0\"},{\"symbol\":\"BLZUSDT\",\"initialMargin\":\"0\",\"maintMargin\":\"0\",\"unrealizedProfit\":\"0.00000000\",\"positionInitialMargin\":\"0\",\"openOrderInitialMargin\":\"0\",\"leverage\":\"20\",\"isolated\":false,\"entryPrice\":\"0.0\",\"maxNotional\":\"25000\",\"positionSide\":\"BOTH\",\"positionAmt\":\"0\",\"notional\":\"0\",\"isolatedWallet\":\"0\",\"updateTime\":0,\"bidNotional\":\"0\",\"askNotional\":\"0\"},{\"symbol\":\"ETHUSDT_220930\",\"initialMargin\":\"0\",\"maintMargin\":\"0\",\"unrealizedProfit\":\"0.00000000\",\"positionInitialMargin\":\"0\",\"openOrderInitialMargin\":\"0\",\"leverage\":\"20\",\"isolated\":false,\"entryPrice\":\"0.0\",\"maxNotional\":\"375000\",\"positionSide\":\"BOTH\",\"positionAmt\":\"0.000\",\"notional\":\"0\",\"isolatedWallet\":\"0\",\"updateTime\":0,\"bidNotional\":\"0\",\"askNotional\":\"0\"},{\"symbol\":\"GMTUSDT\",\"initialMargin\":\"0\",\"maintMargin\":\"0\",\"unrealizedProfit\":\"0.00000000\",\"positionInitialMargin\":\"0\",\"openOrderInitialMargin\":\"0\",\"leverage\":\"20\",\"isolated\":false,\"entryPrice\":\"0.0\",\"maxNotional\":\"150000\",\"positionSide\":\"BOTH\",\"positionAmt\":\"0\",\"notional\":\"0\",\"isolatedWallet\":\"0\",\"updateTime\":0,\"bidNotional\":\"0\",\"askNotional\":\"0\"},{\"symbol\":\"FTMUSDT\",\"initialMargin\":\"0\",\"maintMargin\":\"0\",\"unrealizedProfit\":\"0.00000000\",\"positionInitialMargin\":\"0\",\"openOrderInitialMargin\":\"0\",\"leverage\":\"20\",\"isolated\":false,\"entryPrice\":\"0.0\",\"maxNotional\":\"150000\",\"positionSide\":\"BOTH\",\"positionAmt\":\"0\",\"notional\":\"0\",\"isolatedWallet\":\"0\",\"updateTime\":0,\"bidNotional\":\"0\",\"askNotional\":\"0\"},{\"symbol\":\"1000SHIBBUSD\",\"initialMargin\":\"0\",\"maintMargin\":\"0\",\"unrealizedProfit\":\"0.00000000\",\"positionInitialMargin\":\"0\",\"openOrderInitialMargin\":\"0\",\"leverage\":\"20\",\"isolated\":false,\"entryPrice\":\"0.0\",\"maxNotional\":\"25000\",\"positionSide\":\"BOTH\",\"positionAmt\":\"0\",\"notional\":\"0\",\"isolatedWallet\":\"0\",\"updateTime\":0,\"bidNotional\":\"0\",\"askNotional\":\"0\"},{\"symbol\":\"BANDUSDT\",\"initialMargin\":\"0\",\"maintMargin\":\"0\",\"unrealizedProfit\":\"0.00000000\",\"positionInitialMargin\":\"0\",\"openOrderInitialMargin\":\"0\",\"leverage\":\"20\",\"isolated\":false,\"entryPrice\":\"0.0\",\"maxNotional\":\"25000\",\"positionSide\":\"BOTH\",\"positionAmt\":\"0.0\",\"notional\":\"0\",\"isolatedWallet\":\"0\",\"updateTime\":0,\"bidNotional\":\"0\",\"askNotional\":\"0\"},{\"symbol\":\"XRPBUSD\",\"initialMargin\":\"0\",\"maintMargin\":\"0\",\"unrealizedProfit\":\"0.00000000\",\"positionInitialMargin\":\"0\",\"openOrderInitialMargin\":\"0\",\"leverage\":\"20\",\"isolated\":false,\"entryPrice\":\"0.0\",\"maxNotional\":\"100000\",\"positionSide\":\"BOTH\",\"positionAmt\":\"0.0\",\"notional\":\"0\",\"isolatedWallet\":\"0\",\"updateTime\":0,\"bidNotional\":\"0\",\"askNotional\":\"0\"},{\"symbol\":\"DOGEBUSD\",\"initialMargin\":\"0\",\"maintMargin\":\"0\",\"unrealizedProfit\":\"0.00000000\",\"positionInitialMargin\":\"0\",\"openOrderInitialMargin\":\"0\",\"leverage\":\"20\",\"isolated\":false,\"entryPrice\":\"0.0\",\"maxNotional\":\"100000\",\"positionSide\":\"BOTH\",\"positionAmt\":\"0\",\"notional\":\"0\",\"isolatedWallet\":\"0\",\"updateTime\":0,\"bidNotional\":\"0\",\"askNotional\":\"0\"},{\"symbol\":\"XRPUSDT\",\"initialMargin\":\"0\",\"maintMargin\":\"0\",\"unrealizedProfit\":\"0.00000000\",\"positionInitialMargin\":\"0\",\"openOrderInitialMargin\":\"0\",\"leverage\":\"50\",\"isolated\":true,\"entryPrice\":\"0.0\",\"maxNotional\":\"50000\",\"positionSide\":\"BOTH\",\"positionAmt\":\"0.0\",\"notional\":\"0\",\"isolatedWallet\":\"0\",\"updateTime\":1653480562515,\"bidNotional\":\"0\",\"askNotional\":\"0\"},{\"symbol\":\"FTTUSDT\",\"initialMargin\":\"0\",\"maintMargin\":\"0\",\"unrealizedProfit\":\"0.00000000\",\"positionInitialMargin\":\"0\",\"openOrderInitialMargin\":\"0\",\"leverage\":\"20\",\"isolated\":false,\"entryPrice\":\"0.0\",\"maxNotional\":\"25000\",\"positionSide\":\"BOTH\",\"positionAmt\":\"0.0\",\"notional\":\"0\",\"isolatedWallet\":\"0\",\"updateTime\":0,\"bidNotional\":\"0\",\"askNotional\":\"0\"},{\"symbol\":\"SXPUSDT\",\"initialMargin\":\"0\",\"maintMargin\":\"0\",\"unrealizedProfit\":\"0.00000000\",\"positionInitialMargin\":\"0\",\"openOrderInitialMargin\":\"0\",\"leverage\":\"20\",\"isolated\":false,\"entryPrice\":\"0.0\",\"maxNotional\":\"25000\",\"positionSide\":\"BOTH\",\"positionAmt\":\"0.0\",\"notional\":\"0\",\"isolatedWallet\":\"0\",\"updateTime\":0,\"bidNotional\":\"0\",\"askNotional\":\"0\"},{\"symbol\":\"CRVUSDT\",\"initialMargin\":\"0\",\"maintMargin\":\"0\",\"unrealizedProfit\":\"0.00000000\",\"positionInitialMargin\":\"0\",\"openOrderInitialMargin\":\"0\",\"leverage\":\"20\",\"isolated\":false,\"entryPrice\":\"0.0\",\"maxNotional\":\"150000\",\"positionSide\":\"BOTH\",\"positionAmt\":\"0.0\",\"notional\":\"0\",\"isolatedWallet\":\"0\",\"updateTime\":0,\"bidNotional\":\"0\",\"askNotional\":\"0\"},{\"symbol\":\"BELUSDT\",\"initialMargin\":\"0\",\"maintMargin\":\"0\",\"unrealizedProfit\":\"0.00000000\",\"positionInitialMargin\":\"0\",\"openOrderInitialMargin\":\"0\",\"leverage\":\"20\",\"isolated\":false,\"entryPrice\":\"0.0\",\"maxNotional\":\"25000\",\"positionSide\":\"BOTH\",\"positionAmt\":\"0\",\"notional\":\"0\",\"isolatedWallet\":\"0\",\"updateTime\":0,\"bidNotional\":\"0\",\"askNotional\":\"0\"},{\"symbol\":\"DOTUSDT\",\"initialMargin\":\"0\",\"maintMargin\":\"0\",\"unrealizedProfit\":\"0.00000000\",\"positionInitialMargin\":\"0\",\"openOrderInitialMargin\":\"0\",\"leverage\":\"3\",\"isolated\":true,\"entryPrice\":\"0.0\",\"maxNotional\":\"10000000\",\"positionSide\":\"BOTH\",\"positionAmt\":\"0.0\",\"notional\":\"0\",\"isolatedWallet\":\"0\",\"updateTime\":1638379357219,\"bidNotional\":\"0\",\"askNotional\":\"0\"},{\"symbol\":\"XEMUSDT\",\"initialMargin\":\"0\",\"maintMargin\":\"0\",\"unrealizedProfit\":\"0.00000000\",\"positionInitialMargin\":\"0\",\"openOrderInitialMargin\":\"0\",\"leverage\":\"20\",\"isolated\":false,\"entryPrice\":\"0.0\",\"maxNotional\":\"25000\",\"positionSide\":\"BOTH\",\"positionAmt\":\"0\",\"notional\":\"0\",\"isolatedWallet\":\"0\",\"updateTime\":0,\"bidNotional\":\"0\",\"askNotional\":\"0\"},{\"symbol\":\"GMTBUSD\",\"initialMargin\":\"0\",\"maintMargin\":\"0\",\"unrealizedProfit\":\"0.00000000\",\"positionInitialMargin\":\"0\",\"openOrderInitialMargin\":\"0\",\"leverage\":\"20\",\"isolated\":false,\"entryPrice\":\"0.0\",\"maxNotional\":\"25000\",\"positionSide\":\"BOTH\",\"positionAmt\":\"0.0\",\"notional\":\"0\",\"isolatedWallet\":\"0\",\"updateTime\":0,\"bidNotional\":\"0\",\"askNotional\":\"0\"},{\"symbol\":\"ONEUSDT\",\"initialMargin\":\"0\",\"maintMargin\":\"0\",\"unrealizedProfit\":\"0.00000000\",\"positionInitialMargin\":\"0\",\"openOrderInitialMargin\":\"0\",\"leverage\":\"20\",\"isolated\":false,\"entryPrice\":\"0.0\",\"maxNotional\":\"25000\",\"positionSide\":\"BOTH\",\"positionAmt\":\"0\",\"notional\":\"0\",\"isolatedWallet\":\"0\",\"updateTime\":0,\"bidNotional\":\"0\",\"askNotional\":\"0\"},{\"symbol\":\"1000LUNCBUSD\",\"initialMargin\":\"0\",\"maintMargin\":\"0\",\"unrealizedProfit\":\"0.00000000\",\"positionInitialMargin\":\"0\",\"openOrderInitialMargin\":\"0\",\"leverage\":\"20\",\"isolated\":false,\"entryPrice\":\"0.0\",\"maxNotional\":\"25000\",\"positionSide\":\"BOTH\",\"positionAmt\":\"0\",\"notional\":\"0\",\"isolatedWallet\":\"0\",\"updateTime\":0,\"bidNotional\":\"0\",\"askNotional\":\"0\"},{\"symbol\":\"ZILUSDT\",\"initialMargin\":\"0\",\"maintMargin\":\"0\",\"unrealizedProfit\":\"0.00000000\",\"positionInitialMargin\":\"0\",\"openOrderInitialMargin\":\"0\",\"leverage\":\"20\",\"isolated\":false,\"entryPrice\":\"0.0\",\"maxNotional\":\"25000\",\"positionSide\":\"BOTH\",\"positionAmt\":\"0\",\"notional\":\"0\",\"isolatedWallet\":\"0\",\"updateTime\":0,\"bidNotional\":\"0\",\"askNotional\":\"0\"},{\"symbol\":\"AXSUSDT\",\"initialMargin\":\"0\",\"maintMargin\":\"0\",\"unrealizedProfit\":\"0.00000000\",\"positionInitialMargin\":\"0\",\"openOrderInitialMargin\":\"0\",\"leverage\":\"20\",\"isolated\":false,\"entryPrice\":\"0.0\",\"maxNotional\":\"250000\",\"positionSide\":\"BOTH\",\"positionAmt\":\"0\",\"notional\":\"0\",\"isolatedWallet\":\"0\",\"updateTime\":0,\"bidNotional\":\"0\",\"askNotional\":\"0\"},{\"symbol\":\"DYDXUSDT\",\"initialMargin\":\"0\",\"maintMargin\":\"0\",\"unrealizedProfit\":\"0.00000000\",\"positionInitialMargin\":\"0\",\"openOrderInitialMargin\":\"0\",\"leverage\":\"20\",\"isolated\":false,\"entryPrice\":\"0.0\",\"maxNotional\":\"150000\",\"positionSide\":\"BOTH\",\"positionAmt\":\"0.0\",\"notional\":\"0\",\"isolatedWallet\":\"0\",\"updateTime\":0,\"bidNotional\":\"0\",\"askNotional\":\"0\"},{\"symbol\":\"OCEANUSDT\",\"initialMargin\":\"0\",\"maintMargin\":\"0\",\"unrealizedProfit\":\"0.00000000\",\"positionInitialMargin\":\"0\",\"openOrderInitialMargin\":\"0\",\"leverage\":\"20\",\"isolated\":false,\"entryPrice\":\"0.0\",\"maxNotional\":\"25000\",\"positionSide\":\"BOTH\",\"positionAmt\":\"0\",\"notional\":\"0\",\"isolatedWallet\":\"0\",\"updateTime\":0,\"bidNotional\":\"0\",\"askNotional\":\"0\"},{\"symbol\":\"LEVERBUSD\",\"initialMargin\":\"0\",\"maintMargin\":\"0\",\"unrealizedProfit\":\"0.00000000\",\"positionInitialMargin\":\"0\",\"openOrderInitialMargin\":\"0\",\"leverage\":\"20\",\"isolated\":false,\"entryPrice\":\"0.0\",\"maxNotional\":\"25000\",\"positionSide\":\"BOTH\",\"positionAmt\":\"0\",\"notional\":\"0\",\"isolatedWallet\":\"0\",\"updateTime\":0,\"bidNotional\":\"0\",\"askNotional\":\"0\"},{\"symbol\":\"CHZUSDT\",\"initialMargin\":\"0\",\"maintMargin\":\"0\",\"unrealizedProfit\":\"0.00000000\",\"positionInitialMargin\":\"0\",\"openOrderInitialMargin\":\"0\",\"leverage\":\"3\",\"isolated\":true,\"entryPrice\":\"0.0\",\"maxNotional\":\"250000\",\"positionSide\":\"BOTH\",\"positionAmt\":\"0\",\"notional\":\"0\",\"isolatedWallet\":\"0\",\"updateTime\":1638371954905,\"bidNotional\":\"0\",\"askNotional\":\"0\"},{\"symbol\":\"ANKRUSDT\",\"initialMargin\":\"0\",\"maintMargin\":\"0\",\"unrealizedProfit\":\"0.00000000\",\"positionInitialMargin\":\"0\",\"openOrderInitialMargin\":\"0\",\"leverage\":\"20\",\"isolated\":false,\"entryPrice\":\"0.0\",\"maxNotional\":\"25000\",\"positionSide\":\"BOTH\",\"positionAmt\":\"0\",\"notional\":\"0\",\"isolatedWallet\":\"0\",\"updateTime\":0,\"bidNotional\":\"0\",\"askNotional\":\"0\"},{\"symbol\":\"DUSKUSDT\",\"initialMargin\":\"0\",\"maintMargin\":\"0\",\"unrealizedProfit\":\"0.00000000\",\"positionInitialMargin\":\"0\",\"openOrderInitialMargin\":\"0\",\"leverage\":\"20\",\"isolated\":false,\"entryPrice\":\"0.0\",\"maxNotional\":\"25000\",\"positionSide\":\"BOTH\",\"positionAmt\":\"0\",\"notional\":\"0\",\"isolatedWallet\":\"0\",\"updateTime\":0,\"bidNotional\":\"0\",\"askNotional\":\"0\"},{\"symbol\":\"CTSIUSDT\",\"initialMargin\":\"0\",\"maintMargin\":\"0\",\"unrealizedProfit\":\"0.00000000\",\"positionInitialMargin\":\"0\",\"openOrderInitialMargin\":\"0\",\"leverage\":\"20\",\"isolated\":false,\"entryPrice\":\"0.0\",\"maxNotional\":\"25000\",\"positionSide\":\"BOTH\",\"positionAmt\":\"0\",\"notional\":\"0\",\"isolatedWallet\":\"0\",\"updateTime\":0,\"bidNotional\":\"0\",\"askNotional\":\"0\"}]}"
  n1 = case shown="No Error" "error in (no error)" {
    selector: "error in (no error)" -> [w13 w24]
    tunnel: [w10 w24] -> w5
    tunnel: [w14 w23] -> w1
    tunnel: "BinanceAPI in" -> [w18 w23]
    tunnel: [w9 "Error" ("Dane")] -> w4
    tunnel: [w7 _] -> w3
    frame No Error {
      # "API_BINANCE_Execute_Function.vi"
      n2 = Bundle By Name(cluster=w18, "API_FUNCTION"="/fapi/v2/account", "IS_SHA256_NEEDED?"=TRUE, "IS_PARAMETERS?"=FALSE, "API_ENDPOINT_KIND"=enum16{"POST", "DELETE", "GET", "PUT"}."GET", "IS_TIMESTEP_NEEDED"=TRUE, "API_BASE_ENDPOINT_KIND"=T2."USDT_FUTURES") -> (w15:refnum<class "BinanceAPI_.lvclass">)
      n3 = call "API_BINANCE_Execute_Function.vi"("BinanceAPI in"=w15, "error in (no error)"=w13) -> ("BinanceAPI out"=w14:refnum<class "BinanceAPI_.lvclass">, "Body"=w9:string, "error out"=w11:errorcluster)  [unwired: 9 in, 2 out]
      n4 = Unflatten From JSON(JSON string=w9, type and defaults=T1 {"feeTier"=0.0, "canTrade"=TRUE, "canDeposit"=TRUE, "canWithdraw"=TRUE, "updateTime"=0.0, "totalInitialMargin"="", "totalMaintMargin"="", "totalWalletBalance"="", "totalUnrealizedProfit"="", "totalMarginBalance"="", "totalPositionInitialMargin"="", "totalOpenOrderInitialMargin"="", "totalCrossWalletBalance"="", "totalCrossUnPnl"="", "availableBalance"="", "maxWithdrawAmount"="", "assets"=[], "positions"=[]}, error in (no error)=w11) -> (value=w7:T1, error out=w10:errorcluster)  [unwired: 4 in]
    }
    frame Error {
    }
  }
  "error out" <- w5
  "Data" <- w4
  "data" <- w3
  "BinanceAPI out" <- w1
